vi "Text control 2 v4.5_pump-specific.vi"() -> ()   [LabVIEW 2016]
panel:
  in  "Tab Control":enum32{"Main", "Other parameters"}(tab)
  out "Line running":i32
  out "Total lines":i32
  out "Path":path=path "C:/users/rlp38/09Apr2009LTtesting/test2.txt"
  out "I vs Vg":cluster{"Y data in":dbl[], "X data in":dbl[]}[](graph)
  out "Is":dbl format="%.2e"
  out "Id":dbl format="%.2e"
  out "Ig":dbl format="%.2e"
  out "Id max vs time":cluster{"Y data in":dbl[], "X data in":dbl[]}[](graph)
  out "Id min vs time":cluster{"Y data in":dbl[], "X data in":dbl[]}[](graph)
  out "I vs Vd":cluster{"Y data in":dbl[], "X data in":dbl[]}[](graph)
  in  "Program":string="#pulsedstressV d 0.03 20 0 0.5 0.0827 5\n#\n#itime s\n#gaterangemode l\n#drainrangemode l\n#pump /1Q #query pump\n#wait 1000 #wait 1 second\n#pump /1ZR #initialize pump\n#pump /1Q #query pump\n#wait 20000 #wait 20 seconds\n#pump /1N0R #set step resolution: 0.01 mm\n#pump /1Q #query pump\n#wait 1000 #wait 1 second\n#pump /1V300R #choose speed: 300 steps/s\n#pump /1Q #query pump\n#wait 1000 #wait 1 second\n#pump /1O3R #go to port 3, counterclockwise rotation\n#pump /1Q #query pump\n#wait 1000 #wait 1 second\n#pump /1A2400R #go to absolute position 2400\n#pump /1Q #query pump\n#wait 1000 #wait 1 second\n#pump /1Q #query pump\n#pump /1? #report absolute plunger position\n#pump /1V80R #set speed to 80 steps/s\n#pump /1Q #query pump\n#pump /1O5 #switch to port 5, counterclockwise rotation\n#pump /1Q #query pump\n#wait 200 #wait 200 milliseconds\n#pump /1A0R #go to absolute position 0 (= empty syringe)\n#pump /1Q #query pump\n#pump /1? #report absolute plunger position\n#pulsed on 0.05 0 0.02\n#transfer d 1 -1 -0.1 -1 -1 0\n#wait-min 1\n#transfer d 1 -1 -0.1 -1 -1 0\n#output d 0 -1 -0.5 0 -1 -0.1\n#transfer d -10 40 1 5 40 35\n#transfer d -10 40 1 5 40 35\n#output d 0 40 20 0 40 1\n#\n#\n#sample 1 0.008 221 6 0.003\n#samplei 400e-6 200 6 0.002 0.1\n#vsu2pulse -10 4\n#\n#stressV 0.016 0.03 2e-4 0.1e-3 11\n#stressI 220e-7 0.08 15\n#transfer s -1 1 0.5 -0.005 0.005 0.005\n#output s 0 0 0 -0.008 0.008 0.002"
  out "Command running:":string="#output s 0 0 0 -0.008 0.008 0.002"
  out "Serial port data":string
  out "Elapsed Time":dbl caption="Elapsed Time (s)"
  in  "Units":u16(ring) items=["Seconds", "Minutes", "Hours"]
  in  "Time Offset":dbl caption="Set Start Time (s)"
  in  "Reset":bool
  in  "Auto Reset":bool
  in  "integration time":u32(slide) max=2 step=1 scale=0.0..2.0
  in  "Interrupt run":bool
  out "Absolute plunger position vs time":cluster{"Y data in":dbl[], "X data in":dbl[]}[](graph)
  out "Valve position vs time":cluster{"Y data in":dbl[], "X data in":dbl[]}[](graph)
  in  "Halt pump":bool
  in  "Hard stop pump":bool
  in  "Gate Range\nmode":u16(ring) items=["Auto", "Limited", "Fixed"]
  in  "Gate Range":u8(slide)=6 max=11 scale=0.0..11.0
  in  "Source/Drain\nRange mode":u16(ring) items=["Auto", "Limited", "Fixed"]
  in  "Source/Drain Range":u8(slide)=6 max=11 scale=0.0..11.0
  in  "Panel Controls":T1={"Emergency Stop"=refnum, "TransGraph Max"=1e-05, "Text/Graph (text=false)"=TRUE} {"TransGraph Max" format="%.2e"}
  in  "Panel Controls 2":T2={"Emergency Stop"=refnum, "TransGraph Max"=1e-05, "Text/Graph (text=false)"=TRUE, "TransGraph Min"=1e-11} {"TransGraph Min" format="%.2e"; "TransGraph Max" format="%.2e"}
  in  "SMU4":cluster{"on/off":bool, "Voltage":dbl} {"Voltage" min=-100.0 max=100.0 format="%.2f"}
  in  "Full Reset":bool
  in  "Standby":T3
  out "error out":errorcluster
  in  "Delay before read (ms)":u32=1000
  in  "byte count":u32=64
  in  "Serial End Mode for Reads":u16(ring)=2 items=["None", "LastBit", "TermChar"]
  in  "Timeout (ms)":u32=10000
  in  "Enable Termination\nChar (T)":bool=TRUE
  in  "Termination char\n(0xA = '\\n' = LF)\n(0xD = '\\r' = CR)":u8=13 format="%.0x"
  in  "flow control":u16(ring) items=["None"=0, "XON/XOFF"=1, "RTS/CTS"=2, "DTR/DSR"=4]
  in  "stop bits":u16(ring)=10 items=["1.0"=10, "1.5"=15, "2.0"=20]
  in  "parity":u16(ring) items=["None", "Odd", "Even", "Mark", "Space"]
  in  "data bits":u16=8 min=5 max=8 step=1
  in  "VISA resource name":refnum<visa-resource-name>="COM6"
  in  "baud rate":u32=9600
  in  "Drain: Compliance":dbl=0.001 format="%.8f"
  in  "Gate: Compliance":dbl=0.001 format="%.8f"
  in  "hold time /s":dbl format="%.2f"
  in  "delay time /s":dbl format="%.2f"
  in  "Integration time (short)":dbl=0.0019 min=8e-05 max=0.0019 step=8e-05 format="%^.0e"
  in  "Integration time (long)":dbl=0.32 min=0.04 max=2.0 step=0.02 format="%.2f"
  in  "Step delay /s":dbl format="%.2f"
  in  "Prefix (transfer)":string="_step_1_air_"
  in  "Suffix (transfer)":string="_Vg=0_T_1.txt"
  in  "Prefix (time data)":string="_buffer_Idmax_Idmin_vs_time_Vg=-1.0V_Vd=-1.0V"
  in  "Suffix (time data)":string=".txt"
  in  "Prefix (output)":string="_step_1_air_"
  in  "Suffix (output)":string="_Vg=0_O_1.txt"
  in  "Gate":T4={"Gate Start"=0.0, "Gate Stop"=2.0, "Gate Step (linear only)"=1.0, "Gate Compliance"=0.0001, "Gate PComp"=0.0, "Range mode"=0, "Range"=6} {"Range" max=11 scale=0.0..11.0; "Range mode" items=["Auto", "Limited", "Fixed"]; "Gate PComp" format="%^.2e"; "Gate Compliance" format="%^.2e"; "Gate Step (linear only)" format="%^.4e"; "Gate Stop" format="%^.4e"; "Gate Start" format="%^.4e"}
  in  "Drain 2":T5={"Drain Start"=0.0, "Drain Stop"=2.0, "Drain Compliance"=0.0001, "Drain Step"=1.0, "Drain PComp"=0.0, "Range mode"=0, "Range"=6} {"Range" max=11 scale=0.0..11.0; "Range mode" items=["Auto", "Limited", "Fixed"]; "Drain PComp" format="%^.2e"; "Drain Step" format="%^.4e"; "Drain Compliance" format="%^.2e"; "Drain Stop" format="%^.4e"; "Drain Start" format="%^.4e"}
  in  "Timings 2":T6={"integration time"=0, "Short/Long integration time"=0.00064, "hold time (sec)"=0.0, "delay time (sec)"=0.0, "Step Time (0 disables)"=0.0, "sweep method"=0, "Pulse period"=0.005, "Base voltage"=0.0, "Pulse width"=0.0005} {"Pulse width" min=0.0005 max=0.1 step=0.0001 format="%.4f"; "Base voltage" format="%^.4e"; "Pulse period" min=0.005 max=1.0 step=0.0001 format="%.4f"; "sweep method" items=["Continuous", "Pulsed"]; "Step Time (0 disables)" format="%.2f"; "delay time (sec)" format="%.4f"; "hold time (sec)" format="%.4f"; "Short/Long integration time" format="%^.0e"; "integration time" scale=0.0..2.0}
  # "Syntax:\nitime [s|m|l]\ngaterangemode [a|l|f]\ndrainrangemode [a|l|f]\npulsed [on|off] PulsePeriod(sec) PulseBaseVoltage PulseONWidth(sec)\nstandby [on l off]\nwait NumMilliseconds\nwait-min NumMinutes\n# texthere = comment\ntransfer [s|d] VgStart VgStop VgStep VdStart VdStop VdStep\noutput [s|d] VgStart VgStop VgStep VdStart VdStop VdStep\nsample Vg Vd NumSamples Time(s) SampleInterval(s)\nsamplei Idg NumSamples Time(s) SampleInterval(s) VDGcompliance\n100 samples is approximately 13 seconds with medium integration\n# if in doubt use SampleInterval(s) = 0.004\nstressV VG VD IGcompliance IDcompliance Duration(sec)\nstressI IDG VDGcompliance Duration(sec)\nvsu2pulse Bias Duration(s)\npulsedstressV [s|d] VEstop VgON VgOFF Period(s) PulseONwidth(s) Vd\nsample-fpp Vg Vd NumSamples Time\nresample-fpp Vg Vd\ntransfer-fpp [s|d] VgStart VgStop VgStep VdStart VdStop VdStep\noutput-fpp [s|d] VgStart VgStop VgStep VdStart VdStop VdStep\nserial SerialPortCommand\npump SerialPortCommand for the OEM pump\n\nSPM OEM Pump Syntax (<x>: pump number, use 1 if only one pump):\nif the command syntax contains [R], then append the letter R to the command\n/<x>Q: query (a query command should follow each command)\n/<x>Z[R] or /<x>Y[R]: initialize pump\n/<x>N<n>[R] (<n>=0,1): <0> (<1>) microstep 0.01 mm (0.00125 mm) resolution\n/<x>I<n> (<n>=0-6): turn to port number n (clockwise)\n/<x>O<n> (<n>=0-6): turn to port number n (counterclockwise)\n/<x>X: Re-execute last command string\n/<x>G<n>[R] (<n>=0-60000): repeat command sequence (default: 0, 0=loop forever)\n/<x>g: Mark the start of a repeat sequence (max = 10)\n/<x>M<n>[R] (<n>=0-86400000): delay command execution by n milliseconds\n/<x>H: Halt; Pause the sequence after finishing the current move\n/<x>T: Hardstop; Interrupt the current move and suppress it from the sequence\n/<x>A<n>[R] (<n>=0-3000 with N=0, 0-24000 with N=1): absolute position\n/<x>P<n>[R] (<n>=0-3000 with N=0, 0-24000 with N=1): relative pickup\n/<x>D<n>[R] (<n>=0-3000 with N=0, 0-24000 with N=1): relative dispense\n/<x>V<n>[R] (<n>=5-1600 default: 150): set peak speed (pulses/sec)\n/<x>S<n>[R] (<n>=10-40 default: 22): set speed (NOT in pulses/sec, look in manual)\nNOTE: When controlled with absolute position, one does not need to pay special attention to the syringe that is mounted on the pump.\nWithdraw from lower stage (ports 1, 3, 5), dispense from higher stage (ports 2, 4, 6)."
  # "Time"
  # "1\n2\n3\n4\n5\n6\n7\n8\n9\n10\n11\n12\n13\n14\n15\n16\n17\n18\n19\n20"
  # "Serial port settings"
  # "Filename settings"
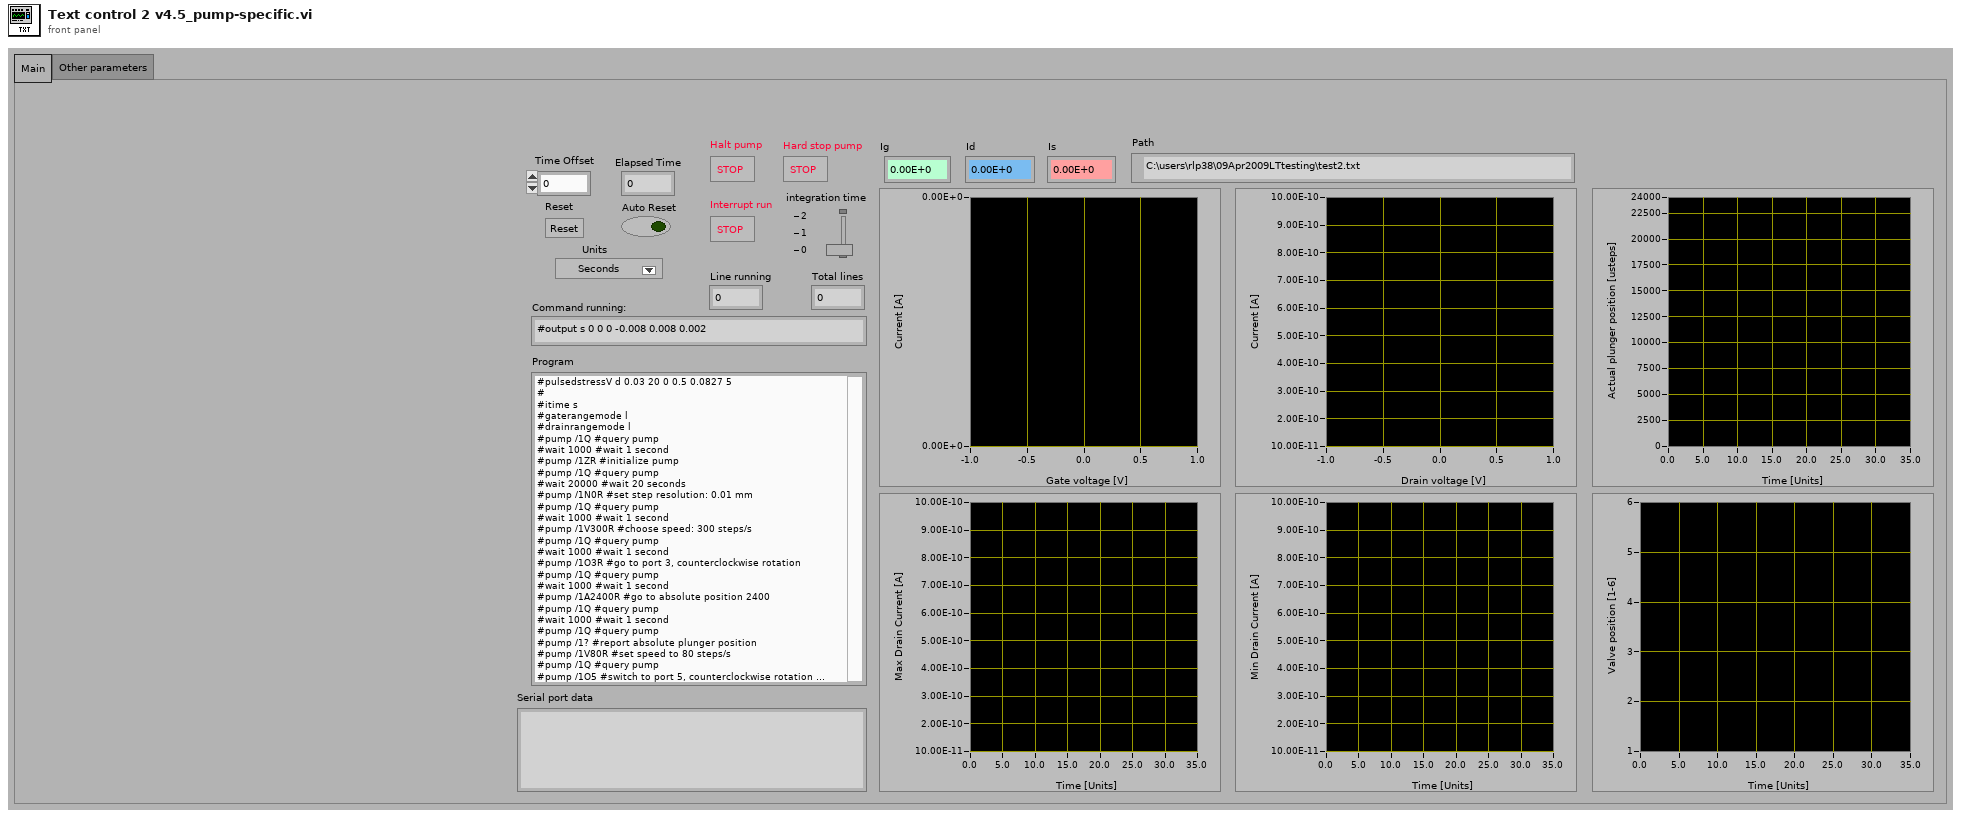
[diagram p1: front panel]
types:
  T1 = cluster{"Emergency Stop":refnum<vi>, "TransGraph Max":dbl, "Text/Graph (text=false)":bool}
  T2 = cluster{"Emergency Stop":refnum<vi>, "TransGraph Max":dbl, "Text/Graph (text=false)":bool, "TransGraph Min":dbl}
  T3 = cluster{"Gate Standby":bool, "Drain Standby":bool}
  T4 = cluster{"Gate Start":dbl, "Gate Stop":dbl, "Gate Step (linear only)":dbl, "Gate Compliance":dbl, "Gate PComp":dbl, "Range mode":u16, "Range":u8}
  T5 = cluster{"Drain Start":dbl, "Drain Stop":dbl, "Drain Compliance":dbl, "Drain Step":dbl, "Drain PComp":dbl, "Range mode":u16, "Range":u8}
  T6 = cluster{"integration time":u32, "Short/Long integration time":dbl, "hold time (sec)":dbl, "delay time (sec)":dbl, "Step Time (0 disables)":dbl, "sweep method":u16, "Pulse period":dbl, "Base voltage":dbl, "Pulse width":dbl}
  T7 = enum16{"open", "replace", "create", "open or create", "replace or create", "replace or create with confirmation"}
  T8 = cluster{"V2 Start":dbl, "V2 Step":dbl, "Number of points":i32}
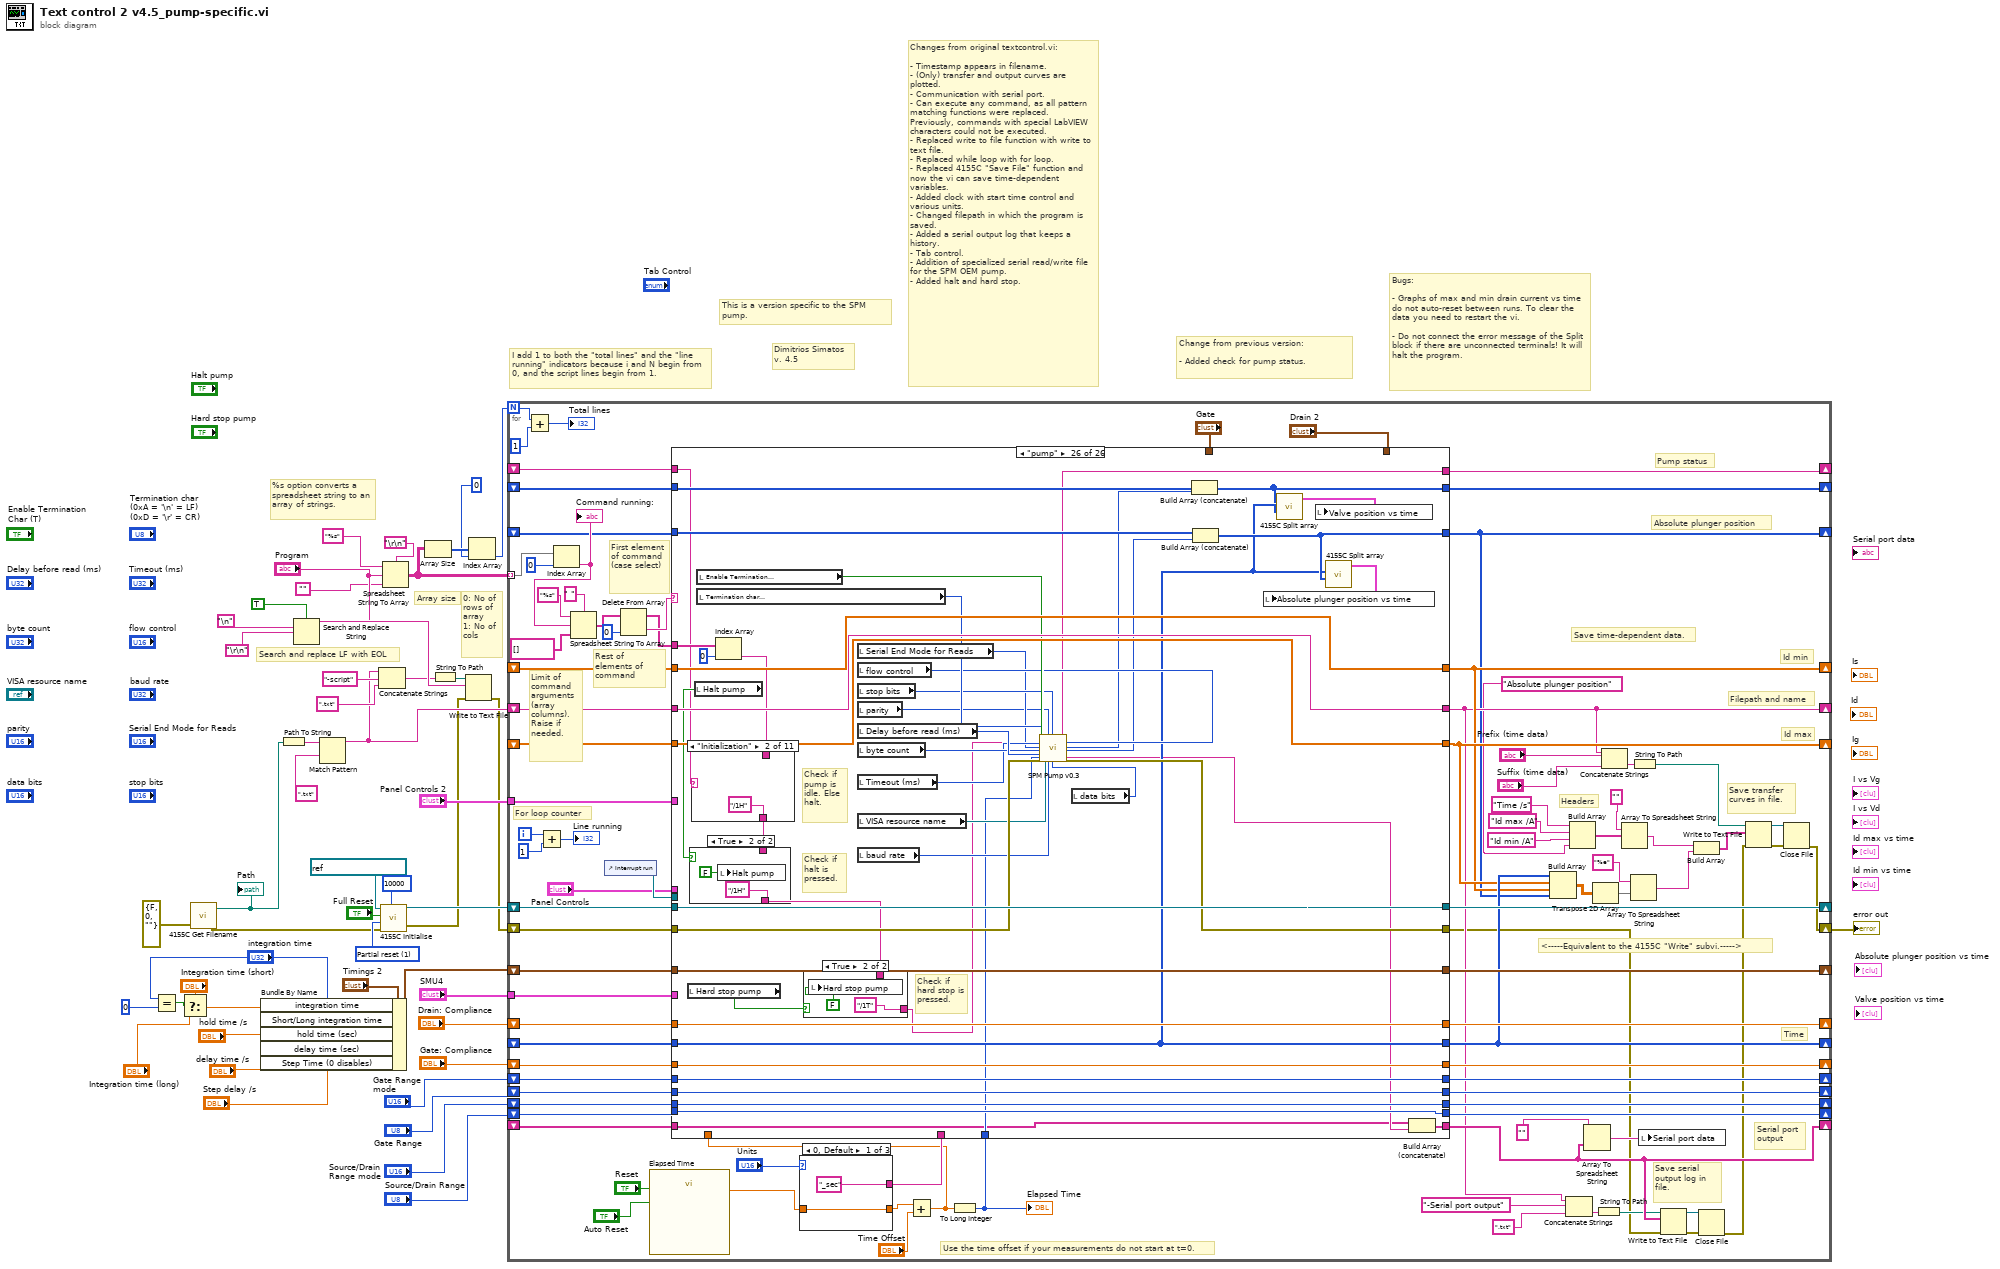
[diagram p0: block diagram]
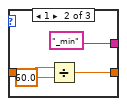
[diagram p2: hidden frame]
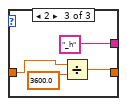
[diagram p3: hidden frame]
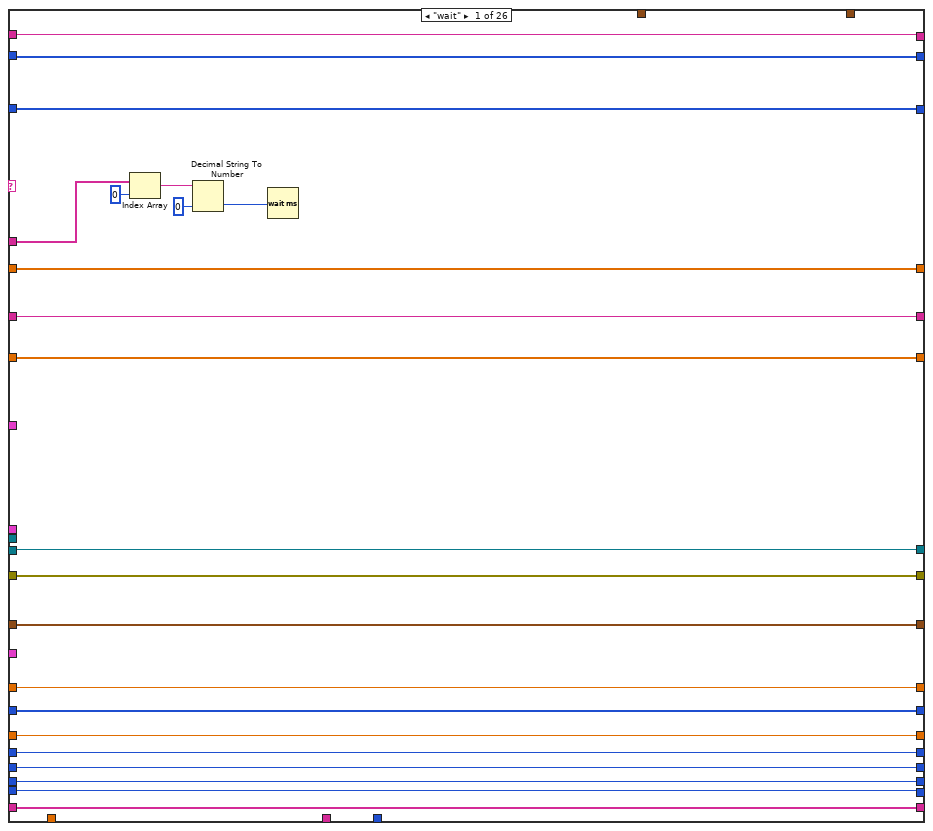
[diagram p4: hidden frame]
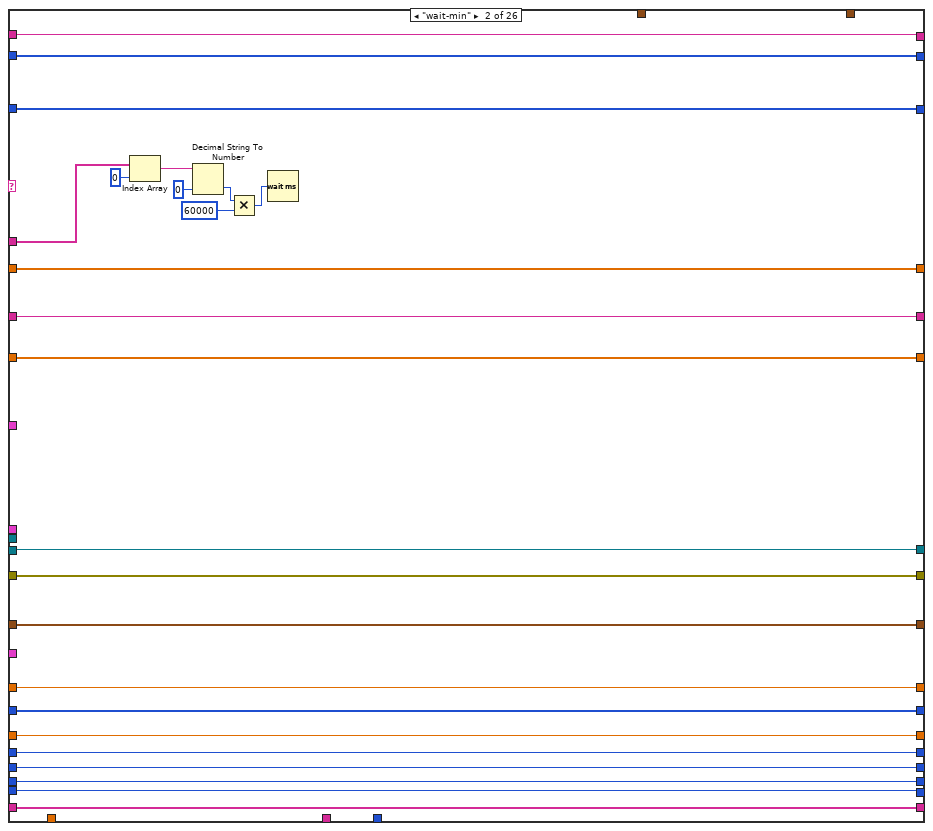
[diagram p5: hidden frame]
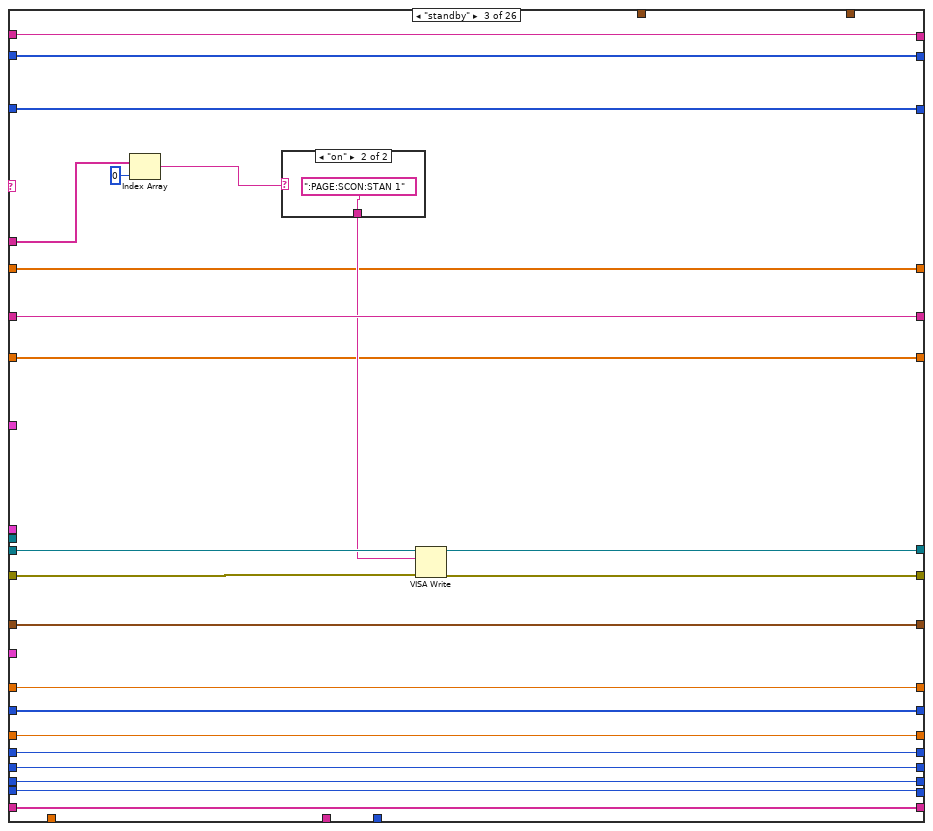
[diagram p6: hidden frame]
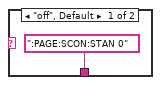
[diagram p7: hidden frame]
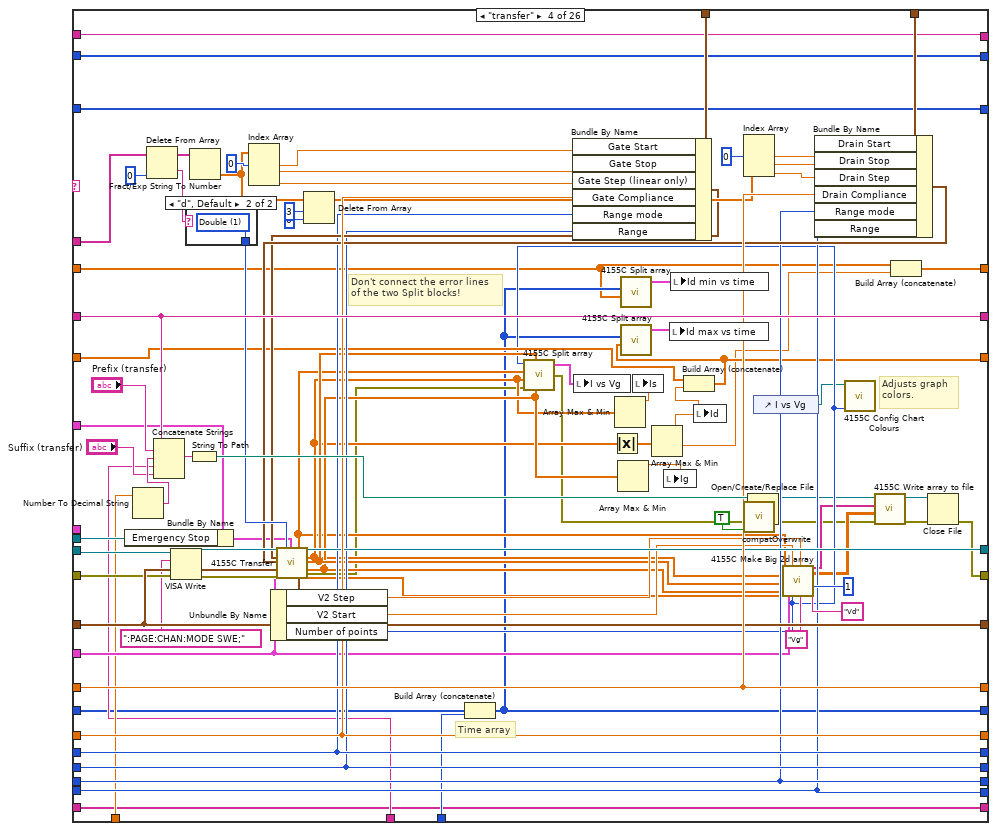
[diagram p8: hidden frame]
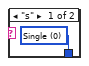
[diagram p9: hidden frame]
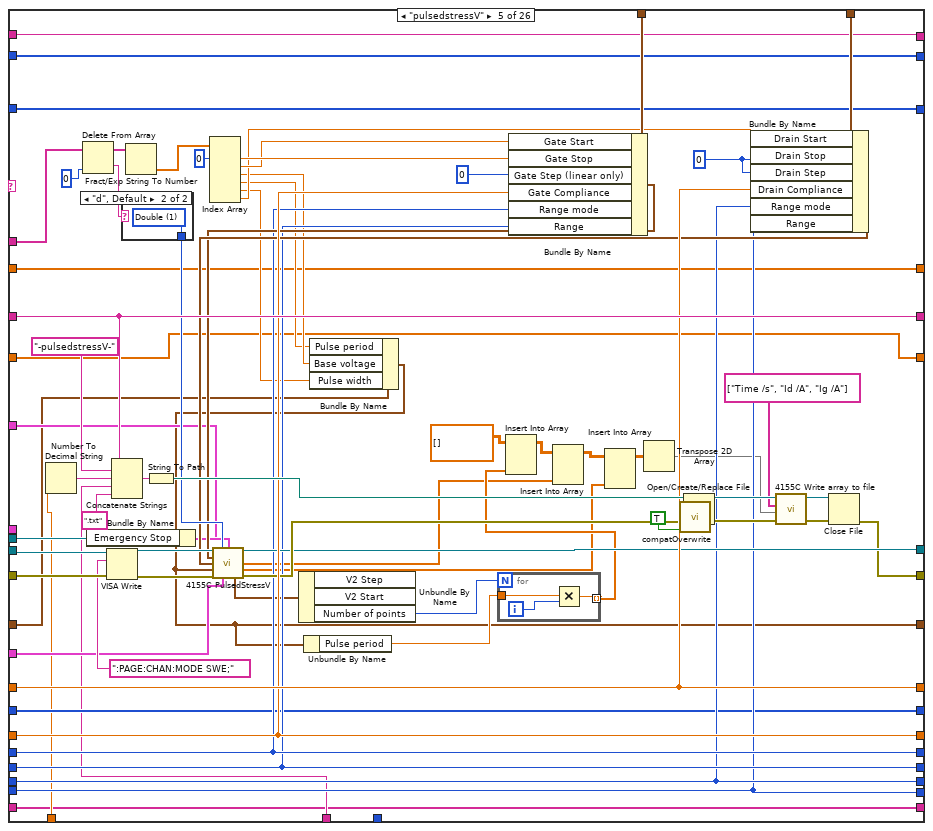
[diagram p10: hidden frame]
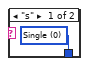
[diagram p11: hidden frame]
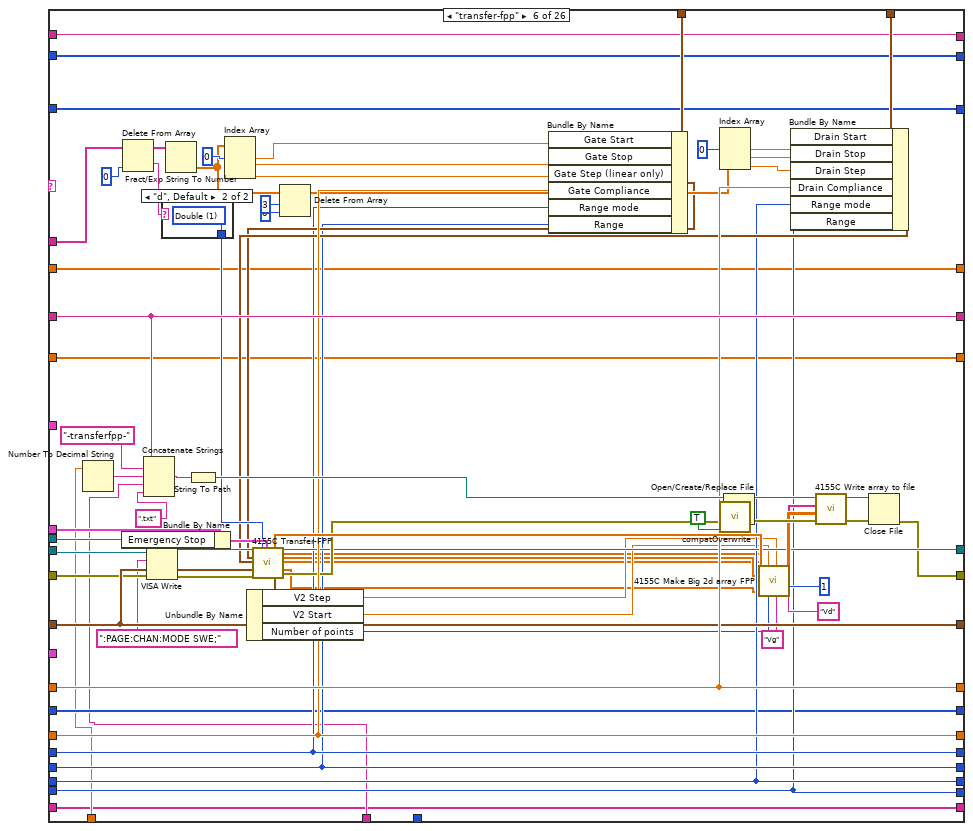
[diagram p12: hidden frame]
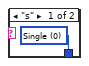
[diagram p13: hidden frame]
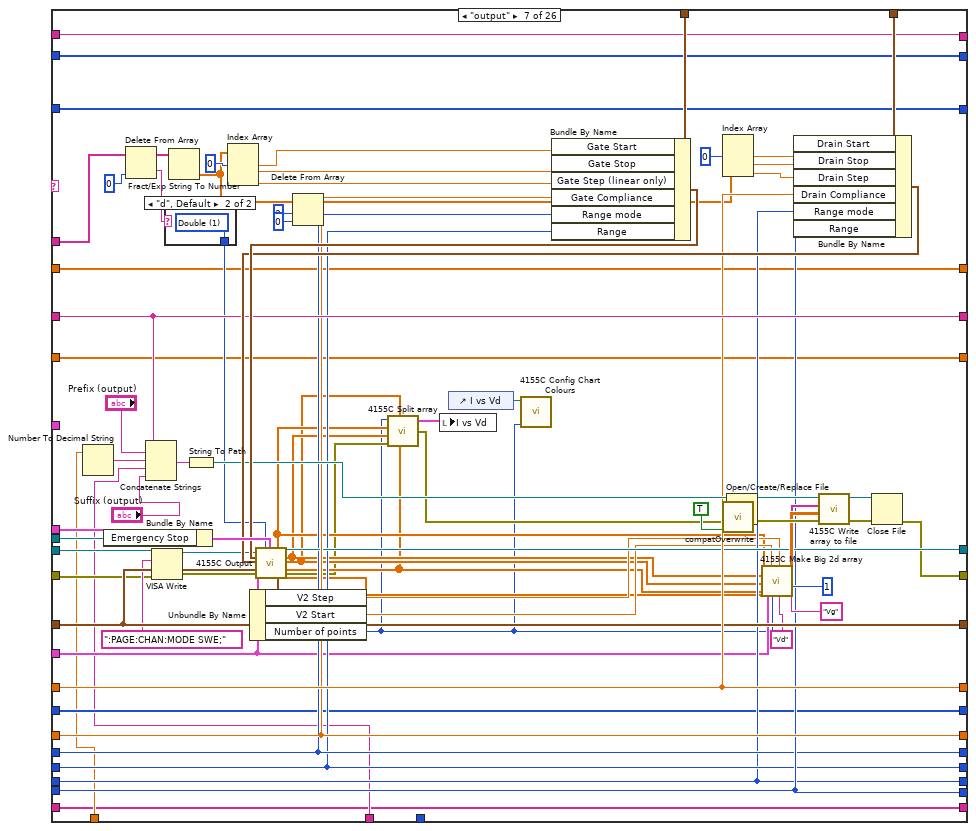
[diagram p14: hidden frame]
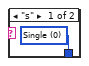
[diagram p15: hidden frame]
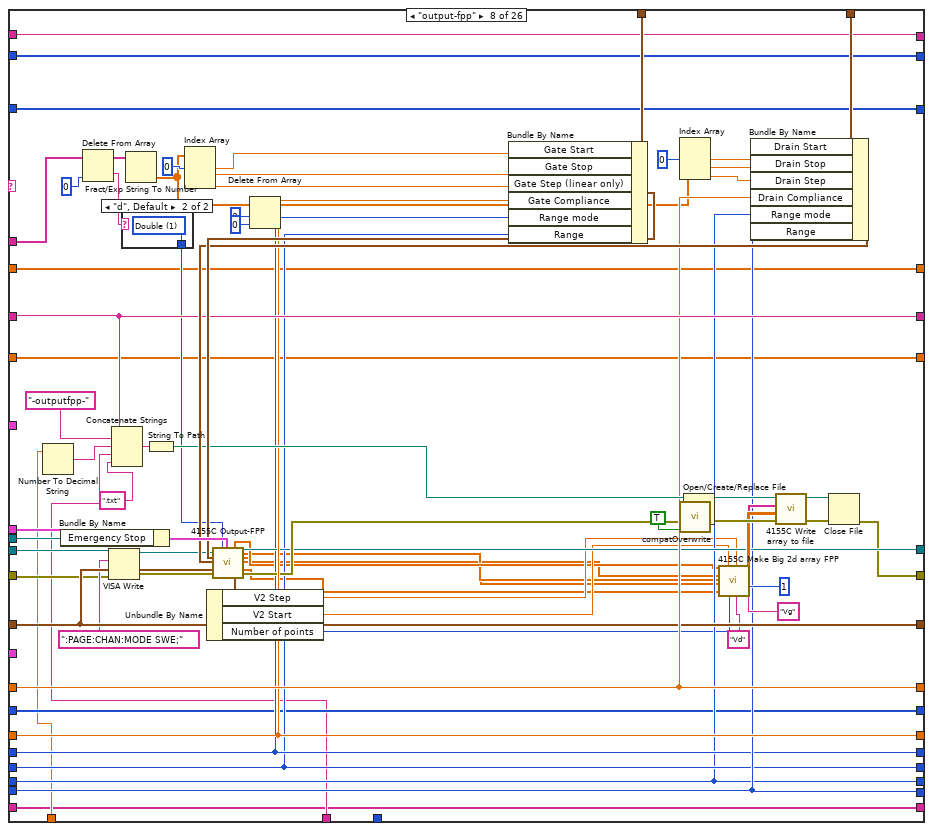
[diagram p16: hidden frame]
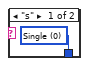
[diagram p17: hidden frame]
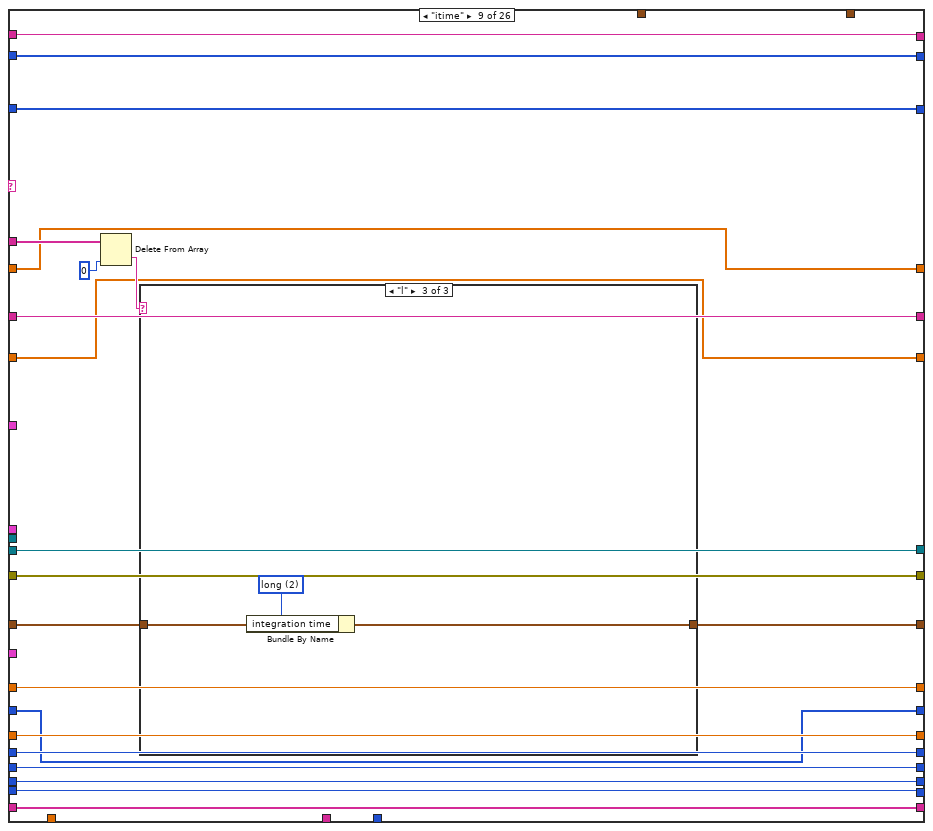
[diagram p18: hidden frame]
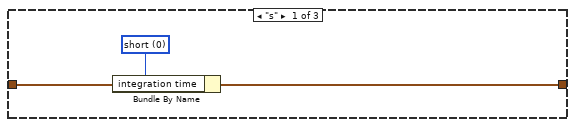
[diagram p19: hidden frame]
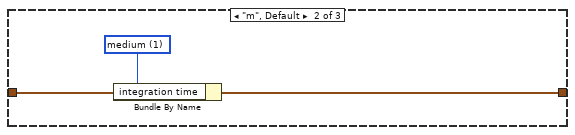
[diagram p20: hidden frame]
diagram:
  w40 = u16 1 items=["Reset All", "Partial reset"] ("Type of reset")
  # "This is a version specific to the SPM pump."
  # "I add 1 to both the \"total lines\" and the \"line running\" indicators because i and N begin from 0, and the script lines begin from 1."
  # "Bugs:\n\n- Graphs of max and min drain current vs time do not auto-reset between runs. To clear the data you need to restart the vi.\n\n- Do not connect the error message of the Split block if there are unconnected terminals! It will halt the program."
  # "Array size"
  # "%s option converts a spreadsheet string to an array of strings."
  # "0: No of rows of array\n1: No of cols"
  # "Change from previous version:\n\n- Added check for pump status."
  # "Dimitrios Simatos\nv. 4.5"
  # "Changes from original textcontrol.vi:\n\n- Timestamp appears in filename.\n- (Only) transfer and output curves are plotted.\n- Communication with serial port.\n- Can execute any command, as all pattern matching functions were replaced. Previously, commands with special LabVIEW characters could not be executed.\n- Replaced write to file function with write to text file.\n- Replaced while loop with for loop.\n- Replaced 4155C \"Save File\" function and now the vi can save time-dependent variables.\n- Added clock with start time control and various units.\n- Changed filepath in which the program is saved.\n- Added a serial output log that keeps a history.\n- Tab control.\n- Addition of specialized serial read/write file for the SPM OEM pump.\n- Added halt and hard stop."
  # "Search and replace LF with EOL"
  n1 = Equal?(x="integration time", y=u32 0) -> (x = y?=w44:bool)
  n2 = Select(t="Integration time (short)", s=w44, f="Integration time (long)") -> (s? t:f=w48:dbl)
  n3 = call "4155C Get Filename.vi"("error in (no error)"=errorcluster {"status"=FALSE, "code"=0, "source"=""}) -> ("error out"=w35:errorcluster, "path"=w10:path)  [unwired: 2 in, 1 out]
  "Path" <- w10
  n4 = Bundle By Name(cluster="Timings 2", "integration time"="integration time", "Short/Long integration time"=w48, "hold time (sec)"="hold time /s", "delay time (sec)"="delay time /s", "Step Time (0 disables)"="Step delay /s") -> (w33:T6)
  n5 = Path To String(path=w10) -> (string=w11:string)
  n6 = Search and Replace String(replace all?=TRUE ("replace all? (F)"), input string="Program", search string="\n", replace string="\r\n") -> (result string=w23:string)  [unwired: 4 in, 3 out]
  n7 = Match Pattern(string=w11, regular expression=".txt") -> (before substring=w5:string)  [unwired: 1 in, 3 out]
  n8 = Concatenate Strings(w5, "-script" ("Prefix"), ".txt" ("regular expression")) -> (w4:string)
  n9 = call "4155C Initialise.vi"("VISA resource name in"=refnum<visa-resource-name> "GPIB0::14::INSTR", "Reset"="Full Reset", "Type of reset"=w40, "error in (no error)"=w35, "VISA Timeout Value"=u32 10000) -> ("VISA Resource Name out"=w34:refnum<visa-resource-name>, "error out"=w2:errorcluster)
  n10 = Spreadsheet String To Array(delimiter (Tab)="\r\n", format string="%s", spreadsheet string="Program", array type (2D Dbl)="") -> (array=w14:string[][])
  n11 = Array Size(array=w14) -> (size(s)=w18:i32[])
  n12 = String To Path(string=w4) -> (path=w3:path)
  n13 = Write to Text File(file (use dialog)=w3, text=w23, error in=w2) -> (error out=w1:errorcluster)  [unwired: 1 in, 2 out]
  n14 = Index Array(array=w18, index=0) -> (element=w16:i32)
  n15 = for {
    N: w16 -> [w75]
    tunnel: "SMU4" -> [w120]
    shift-left: "Source/Drain Range" -> [w125]
    shift-right: [w121] -> _
    shift-left: "Source/Drain\nRange mode" -> [w126]
    shift-right: [w122] -> _
    shift-left: "Gate Range" -> [w127]
    shift-right: [w123] -> _
    shift-left: "Gate Range\nmode" -> [w128]
    shift-right: [w124] -> _
    shift-left: "Gate: Compliance" -> [w137]
    shift-right: [w133] -> _
    shift-left: "Drain: Compliance" -> [w138]
    shift-right: [w134] -> _
    shift-left: w33 -> [w139]
    shift-right: [w135] -> _
    shift-left: w1 -> [w140]
    shift-right: [w83] -> w9
    shift-left: w34 -> [w141]
    shift-right: [w136] -> _
    shift-left: w5 -> [w142]
    shift-right: [w59] -> _
    tunnel: "Panel Controls 2" -> [w119]
    shift-right: [w87] -> _
    shift-left: _ -> [w118]
    shift-right: [w88] -> _
    shift-left: _ -> [w114]
    tunnel: w14 -> [w112] mode=indexing
    shift-right: [w81] -> _
    shift-left: _ -> [w82]
    shift-right: [w64] -> _
    shift-left: _ -> [w67]
    shift-right: [w55] -> _
    shift-left: _ -> [w56]
    shift-right: [w53] -> _
    shift-left: _ -> [w52]
    shift-right: [w51] -> _
    shift-left: _ -> [w50]
    i -> [w70]
    # "Pump status"
    # "Absolute plunger position"
    # "Serial port output"
    # "Save serial output log in file."
    # "For loop counter"
    # "<-----Equivalent to the 4155C \"Write\" subvi.----->"
    # "Headers"
    # "Save transfer curves in file."
    # "Filepath and name"
    # "Save time-dependent data."
    # "Use the time offset if your measurements do not start at t=0."
    # "Time"
    # "Rest of elements of command"
    # "Id min"
    # "Id max"
    # "Limit of command arguments (array columns). Raise if needed."
    # "First element of command\n(case select)"
    n16 = Add(x=w75, y=1) -> (x+y=→"Total lines":i32)
    n17 = Add(x=w70, y=1) -> (x+y=→"Line running":i32)
    n18 = Index Array(array=w112, index=0 ("line index")) -> (element=w107:string)
    "Command running:" <- w107
    n19 = Spreadsheet String To Array(delimiter (Tab)=" ", format string="%s", spreadsheet string=w107, array type (2D Dbl)=string[] []) -> (array=w104:string[])
    n20 = control-ref of="Interrupt run"() -> (w132:refnum<vi>)
    n21 = Delete From Array(array=w104, index=0) -> (deleted portion=w105:string, array with subset deleted=w103:string[])  [unwired: 1 in]
    n22 = call "Elapsed Time"("Reset"="Reset", "Auto Reset"="Auto Reset") -> ("Elapsed Time (s)"=w115:dbl)  [unwired: 10 in, 7 out]
    n23 = case shown="0, Default" "Units" {
      tunnel: ["_sec" "_min" "_h"] -> w116
      tunnel: [w143 w147 w150] -> w77
      tunnel: w115 -> [w143 w146 w151]
      frame 0, Default {
      }
      frame 1 {
        n24 = Divide(x=w146, y=60.0) -> (x/y=w147:dbl)
      }
      frame 2 {
        n25 = Divide(x=w151, y=3600.0) -> (x/y=w150:dbl)
      }
    }
    n26 = Add(x=w77, y="Time Offset") -> (x+y=w76:dbl)
    n27 = To Long Integer(number=w76) -> (32bit integer=w113:i32)
    "Elapsed Time" <- w113
    n28 = case shown="\"pump\"" w105 {
      tunnel: w103 -> [w174 w198 w221 w301 w370 w444 w524 w599 w642 w673 w705 w735 w761 w780 _ _ w899 w965 _ w1040 w1089 w1136 w1211 w1278 w1303 w1352]
      tunnel: w142 -> [w169 w194 w219 w308 w377 w452 w531 w607 w631 w662 w697 w728 w755 w773 w797 w844 w877 w947 w983 w1027 w1076 w1124 w1205 w1274 w1305 w1354]
      tunnel: w141 -> [w168 w193 w210 w279 w361 w421 w500 w575 w632 w663 w698 w729 w756 w774 w802 w846 w905 w971 w987 w1046 w1095 w1142 w1217 w1232 w1309 w1358]
      tunnel: w140 -> [w167 w192 w209 w278 w360 w420 w497 w572 w633 w664 w699 w730 w757 w775 w801 w817 w904 w970 w986 w1045 w1094 w1141 w1216 w1231 w1308 w1357]
      tunnel: w139 -> [w166 w191 w218 w304 w336 w448 w527 w603 w641 w672 w696 w727 w754 w772 w800 w841 w868 w939 w992 w1020 w1069 w1117 w1204 w1273 w1310 w1359]
      tunnel: w138 -> [w165 w190 w217 w306 w375 w450 w529 w605 w640 w671 w704 w734 w760 w779 w799 w826 w903 w969 w995 w1044 w1093 w1140 w1215 w1282 w1311 w1360]
      tunnel: w137 -> [w164 w189 w216 w305 w374 w449 w528 w604 w639 w670 w703 w733 w759 w778 w798 w827 w878 w948 w994 w1028 w1077 w1125 w1206 w1275 w1313 w1361]
      tunnel: [w168 w193 w208 w303 w372 w446 w526 w601 w632 w663 w698 w729 w756 w774 w802 w846 w869 w921 w985 w1021 w1070 w1118 w1157 w1234 w1309 w1358] -> w136
      tunnel: [w167 w192 w207 w302 w371 w445 w525 w600 w633 w664 w699 w730 w757 w775 w801 w816 w879 w922 w984 w1029 w1078 w1126 w1156 w1233 w1307 w1356] -> w58
      tunnel: [w166 w191 w218 w304 w332 w448 w527 w603 w634 w665 w696 w727 w754 w772 w800 w841 w868 w939 w992 w1020 w1069 w1117 w1204 w1273 w1310 w1359] -> w135
      tunnel: [w165 w190 w217 w306 w375 w450 w529 w605 w640 w671 w704 w734 w760 w779 w799 w826 w903 w969 w995 w1044 w1093 w1140 w1215 w1282 w1311 w1360] -> w134
      tunnel: [w164 w189 w216 w305 w374 w449 w528 w604 w639 w670 w703 w733 w759 w778 w798 w827 w878 w948 w994 w1028 w1077 w1125 w1206 w1275 w1313 w1361] -> w133
      tunnel: [w169 w194 w219 w308 w377 w452 w531 w607 w631 w662 w697 w728 w755 w773 w797 w844 w877 w947 w983 w1027 w1076 w1124 w1205 w1274 w1305 w1354] -> w59
      tunnel: w132 -> [_ _ _ w311 w381 w457 w535 w611 _ _ _ _ _ _ _ _ w874 w944 _ w1026 w1075 w1123 w1177 w1250 _ _]
      tunnel: "Gate" -> [_ _ _ w288 w364 w431 w511 w586 _ _ _ _ _ _ _ _ _ _ _ _ _ _ _ _ _ _]
      tunnel: "Drain 2" -> [_ _ _ w287 w363 w430 w510 w585 _ _ _ _ _ _ _ _ _ _ _ _ _ _ _ _ _ _]
      tunnel: "Panel Controls" -> [_ _ _ _ _ w429 w509 w584 _ _ _ _ _ _ _ _ _ _ _ _ _ _ _ _ _ _]
      tunnel: w128 -> [w163 w188 w215 w272 w354 w414 w495 w570 w638 w669 _ w726 w753 w771 w796 w828 w864 w935 w988 w1016 w1065 w1113 w1200 w1269 w1314 w1362]
      tunnel: w127 -> [w162 w187 w214 w271 w353 w413 w494 w569 w637 w668 w702 _ w744 w777 w795 w829 w865 w936 w989 w1017 w1066 w1114 w1201 w1270 w1315 w1363]
      tunnel: w126 -> [w161 w186 w213 w270 w352 w412 w493 w568 w636 w667 w701 w732 w758 _ w794 w830 w866 w937 w990 w1018 w1067 w1115 w1202 w1271 w1316 w1364]
      tunnel: w125 -> [w160 w185 w212 w269 w351 w411 w496 w571 w635 w666 w700 w731 _ w776 w793 w831 w867 w938 w991 w1019 w1068 w1116 w1203 w1272 w1317 w1365]
      tunnel: [w163 w188 w215 w272 w354 w414 w495 w570 w638 w669 w695 w726 w753 w771 w796 w828 w864 w935 w988 w1016 w1065 w1113 w1200 w1269 w1314 w1362] -> w124
      tunnel: [w162 w187 w214 w271 w353 w413 w494 w569 w637 w668 w702 w718 w744 w777 w795 w829 w865 w936 w989 w1017 w1066 w1114 w1201 w1270 w1315 w1363] -> w123
      tunnel: [w161 w186 w213 w270 w352 w412 w493 w568 w636 w667 w701 w732 w758 w770 w794 w830 w866 w937 w990 w1018 w1067 w1115 w1202 w1271 w1316 w1364] -> w122
      tunnel: [w160 w185 w212 w269 w351 w411 w496 w571 w635 w666 w700 w731 w745 w776 w793 w831 w867 w938 w991 w1019 w1068 w1116 w1203 w1272 w1317 w1365] -> w121
      tunnel: w120 -> [_ _ _ w264 w348 _ w489 _ _ _ _ _ _ _ _ _ _ _ _ _ _ _ _ _ _ _]
      tunnel: w119 -> [_ _ _ w262 w347 _ _ _ _ _ _ _ _ _ _ _ _ _ _ _ _ _ _ _ _ _]
      tunnel: [w159 w181 w205 w239 w324 w401 w486 w557 w630 w660 w694 w717 w743 w769 w792 w812 w856 w919 w982 w1005 w1058 w1107 w1154 w1227 w1306 w1355] -> w87
      tunnel: w118 -> [w159 w181 w205 w253 w324 w401 w486 w557 w630 w660 w694 w717 w743 w769 w792 w812 w856 w919 w982 w1005 w1058 w1107 w1154 w1227 w1306 w1355]
      tunnel: w76 -> [_ _ _ w249 w321 w399 w483 w554 _ _ _ _ _ _ _ w810 w854 w916 _ w1002 w1055 w1104 w1151 w1223 _ _]
      tunnel: w116 -> [_ _ _ w246 w320 w397 w482 w553 _ _ _ _ _ _ _ w808 w852 w915 _ w1001 w1054 w1103 w1150 w1224 _ _]
      tunnel: w113 -> [_ _ _ w240 _ _ _ _ _ _ _ _ _ _ _ _ _ _ _ _ _ _ _ _ _ w1320]
      tunnel: [w158 w180 w204 w237 w323 w400 w485 w556 w629 w659 w693 w716 w742 w768 w791 w811 w855 w918 w981 w1004 w1057 w1106 w1153 w1226 w1312 w1334] -> w88
      tunnel: w114 -> [w158 w180 w204 w245 w323 w400 w485 w556 w629 w659 w693 w716 w742 w768 w791 w811 w855 w918 w981 w1004 w1057 w1106 w1153 w1226 w1312 w1334]
      tunnel: [w157 w179 w203 w235 w319 w396 w481 w552 w628 w658 w692 w715 w741 w767 w790 w807 w851 w914 w980 w1000 w1053 w1102 w1149 w1222 w1301 w1351] -> w81
      tunnel: w82 -> [w157 w179 w203 w234 w319 w396 w481 w552 w628 w658 w692 w715 w741 w767 w790 w807 w851 w914 w980 w1000 w1053 w1102 w1149 w1222 w1301 w1351]
      tunnel: [w156 w178 w202 w227 w318 w395 w471 w551 w627 w657 w691 w714 w740 w766 w789 w806 w850 w913 w979 w999 w1052 w1101 w1148 w1221 w1300 w1350] -> w64
      tunnel: w67 -> [w156 w178 w202 w227 w318 w395 w471 w551 w627 w657 w691 w714 w740 w766 w789 w806 w850 w913 w979 w999 w1052 w1101 w1148 w1221 w1299 w1318]
      tunnel: [w155 w177 w201 w226 w317 w394 w470 w550 w626 w656 w690 w713 w739 w765 w788 w805 w849 w912 w978 w998 w1051 w1100 w1147 w1220 w1285 w1336] -> w55
      tunnel: w56 -> [w155 w177 w201 w226 w317 w394 w470 w550 w626 w656 w690 w713 w739 w765 w788 w805 w849 w912 w978 w998 w1051 w1100 w1147 w1220 w1285 w1335]
      tunnel: [w154 w176 w200 w225 w316 w393 w469 w549 w625 w655 w689 w712 w738 w764 w787 w804 w848 w911 w977 w997 w1050 w1099 w1146 w1219 w1284 w1332] -> w53
      tunnel: w52 -> [w154 w176 w200 w225 w316 w393 w469 w549 w625 w655 w689 w712 w738 w764 w787 w804 w848 w911 w977 w997 w1050 w1099 w1146 w1219 w1284 w1331]
      tunnel: [w153 w175 w199 w224 w315 w392 w468 w548 w624 w654 w688 w711 w737 w763 w786 w803 w847 w910 w976 w996 w1049 w1098 w1145 w1218 w1283 w1322] -> w51
      tunnel: w50 -> [w153 w175 w199 w224 w315 w392 w468 w548 w624 w654 w688 w711 w737 w763 w786 w803 w847 w910 w976 w996 w1049 w1098 w1145 w1218 w1283 w1321]
      frame "wait" {
        n29 = Index Array(array=w174, index=0 ("Index")) -> (element=w172:string)
        n30 = Decimal String To Number(string=w172, default (0L)=u32 0) -> (number=w171:u32)  [unwired: 1 in, 1 out]
        n31 = Wait (ms)(milliseconds to wait=w171) -> ()  [unwired: 1 out]
      }
      frame "wait-min" {
        n32 = Index Array(array=w198, index=0 ("Index")) -> (element=w196:string)
        n33 = Decimal String To Number(string=w196, default (0L)=u32 0) -> (number=w184:u32)  [unwired: 1 in, 1 out]
        n34 = Multiply(x=w184, y=u32 60000) -> (x*y=w183:u32)
        n35 = Wait (ms)(milliseconds to wait=w183) -> ()  [unwired: 1 out]
      }
      frame "standby" {
        n36 = Index Array(array=w221, index=0 ("Index")) -> (element=w211:string)
        n37 = case shown="\"on\"" w211 {
          tunnel: [":PAGE:SCON:STAN 0" ":PAGE:SCON:STAN 1"] -> w206
          frame "off", Default {
          }
          frame "on" {
          }
        }
        n38 = VISA Write(VISA resource name=w210, write buffer=w206, error in (no error)=w209) -> (VISA resource name out=w208:refnum<visa-resource-name>, error out=w207:errorcluster)  [unwired: 1 out]
      }
      frame "transfer" {
        # "Don't connect the error lines\nof the two Split blocks!"
        # "Adjusts graph colors."
        # "Time array"
        n39 = Bundle By Name(cluster=w262, "Emergency Stop"=w311) -> (w263:T2)
        n40 = Number To Decimal String(number=w249) -> (decimal integer string=w248:string)  [unwired: 1 in]
        n41 = Delete From Array(array=w301, index=0 ("Index")) -> (deleted portion=w299:string, array with subset deleted=w298:string[])  [unwired: 1 in]
        n42 = Concatenate Strings(w308, "Prefix (transfer)", w248, w246, "Suffix (transfer)") -> (w310:string)
        n43 = VISA Write(VISA resource name=w279, write buffer=":PAGE:CHAN:MODE SWE;" ("write buffer (\"\")"), error in (no error)=w278) -> (VISA resource name out=w276:refnum<visa-resource-name>, error out=w277:errorcluster)  [unwired: 1 out]
        n44 = case shown="\"d\", Default" w299 {
          tunnel: [w313 w314] -> w297
          frame "s" {
            w313 = u16 0 items=["Single", "Double"] ("sweep mode")
          }
          frame "d", Default {
            w314 = u16 1 items=["Single", "Double"] ("sweep mode")
          }
        }
        n45 = String To Path(string=w310) -> (path=w307:path)
        n46 = Fract/Exp String To Number(string=w298) -> (number=w283:dbl[])  [unwired: 3 in, 1 out]
        n47 = Index Array(array=w283, index #1=0 ("Index")) -> (element #1=w296:dbl, element #2=w295:dbl, element #3=w294:dbl)  [unwired: 2 in]
        n48 = Delete From Array(array=w283, length=3 ("Length"), index=0 ("Index")) -> (array with subset deleted=w281:dbl[])  [unwired: 1 out]
        n49 = Build Array (concatenate)(w245, w240) -> (w237:i32[])
        n50 = Bundle By Name(cluster=w288, "Gate Start"=w296, "Gate Stop"=w295, "Gate Step (linear only)"=w294, "Gate Compliance"=w305, "Range mode"=w272, "Range"=w271) -> (w273:T4)
        n51 = call "4155C Split array.vi"("X data in"=w237, "Y1 data in"=w234) -> ("Array of clusters"=w238:cluster{"Y data in":dbl[], "X data in":dbl[]}[])  [unwired: 5 in, 1 out]
        n52 = local write "Id min vs time"(w238) -> ()
        n53 = Index Array(array=w281, index #1=0 ("Index")) -> (element #1=w291:dbl, element #2=w290:dbl, element #3=w289:dbl)  [unwired: 2 in]
        n54 = call <vilib>:"compatOverwrite.vi"("overwrite (F)"=TRUE) -> ("overwrite?"=w261:T7)
        n55 = control-ref of="I vs Vg"() -> (w250:refnum<vi>)
        n56 = Bundle By Name(cluster=w287, "Drain Start"=w291, "Drain Stop"=w290, "Drain Step"=w289, "Drain Compliance"=w306, "Range mode"=w270, "Range"=w269) -> (w274:T5)
        n57 = call "4155C Transfer.vi"("VISA resource name in"=w276, "Gate"=w273, "Drain"=w274, "Timings"=w304, "error in (no error)"=w277, "SMU4"=w264, "sweep mode"=w297, "Panel Controls"=w263) -> ("VG"=w254:dbl[], "Outparams"=w268:T8, "VISA Resource Name out"=w303:refnum<visa-resource-name>, "IS"=w255:dbl[], "ID"=w260:dbl[], "IG"=w256:dbl[], "error out"=w241:errorcluster, "SMU4"=w265:dbl[])  [unwired: 12 in]
        n58 = Unbundle By Name(w268) -> ("V2 Step"=w267:dbl, "V2 Start"=w266:dbl, "Number of points"=w251:i32)
        n59 = call "4155C Split array.vi"("Number of VAR2 steps"=w251, "Y2 data in"=w260, "X data in"=w254, "Y1 data in"=w255, "Y3 data in"=w256, "error in (no error)"=w241) -> ("Array of clusters"=w244:cluster{"Y data in":dbl[], "X data in":dbl[]}[], "error out"=w242:errorcluster)  [unwired: 1 in]
        n60 = local write "I vs Vg"(w244) -> ()
        n61 = Absolute Value(x=w255) -> (abs(x)=w259:dbl[])
        n62 = Array Max & Min(array=w255) -> (max value=w257:dbl)  [unwired: 3 out]
        n63 = Array Max & Min(array=w256) -> (max value=w258:dbl)  [unwired: 3 out]
        n64 = local write "Is"(w257) -> ()
        n65 = Array Max & Min(array=w259) -> (max value=w252:dbl, min value=w236:dbl)  [unwired: 2 out]
        n66 = local write "Ig"(w258) -> ()
        n67 = Build Array (concatenate)(w253, w252) -> (w239:dbl[])
        n68 = call "4155C Split array.vi"("X data in"=w237, "Y1 data in"=w239) -> ("Array of clusters"=w243:cluster{"Y data in":dbl[], "X data in":dbl[]}[])  [unwired: 5 in, 1 out]
        n69 = local write "Id max vs time"(w243) -> ()
        n70 = local write "Id"(w252) -> ()
        n71 = Open/Create/Replace File(file path (use dialog)=w307, error in=w242, operation (0:open)=w261) -> (refnum out=w232:refnum<file>, error out=w230:errorcluster)  [unwired: 3 in, 1 out]
        n72 = call "4155C Make Big 2d array.vi"("1D Var1"=w254, "1d IS"=w255, "1d ID"=w260, "1d IG"=w256, "1d SMU4"=w265, "SMU4"=w264, "VAR2 START"=w266, "Number of VAR2 steps"=w251, "VAR2 STEP"=w267, "VAR1 Name"="Vg", "Decimal places in header"=i8 1, "VAR2 Name"="Vd") -> ("Header array"=w233:string[], "Data array"=w231:dbl[][])  [unwired: 14 in]
        n73 = call "4155C Config Chart Colours.vi"("Numeric"=w251, "XY Graph 2"=w250) -> ()  [unwired: 6 in]
        n74 = call "4155C Write array to file.vi"("Byte Stream File Refnum"=w232, "Header"=w233, "Data Array"=w231, "error in (no error)"=w230) -> ("dup refnum"=w229:refnum<file>, "error out"=w228:errorcluster)  [unwired: 1 in]
        n75 = Build Array (concatenate)(w234, w236) -> (w235:dbl[])
        n76 = Close File(refnum=w229, error in=w228) -> (error out=w302:errorcluster)  [unwired: 1 out]
      }
      frame "pulsedstressV" {
        w330 = 0
        n77 = Number To Decimal String(number=w321) -> (decimal integer string=w378:string)  [unwired: 1 in]
        n78 = Delete From Array(array=w370, index=0 ("Index")) -> (deleted portion=w368:string, array with subset deleted=w367:string[])  [unwired: 1 in]
        n79 = Bundle By Name(cluster=w347, "Emergency Stop"=w381) -> (w349:T2)
        n80 = VISA Write(VISA resource name=w361, write buffer=":PAGE:CHAN:MODE SWE;" ("write buffer (\"\")"), error in (no error)=w360) -> (VISA resource name out=w358:refnum<visa-resource-name>, error out=w359:errorcluster)  [unwired: 1 out]
        n81 = Concatenate Strings(w377, "-pulsedstressV-" ("Substring"), w378, w320, ".txt" ("Substring")) -> (w380:string)
        n82 = case shown="\"d\", Default" w368 {
          tunnel: [w390 w391] -> w366
          frame "s" {
            w390 = u16 0 items=["Single", "Double"] ("sweep mode")
          }
          frame "d", Default {
            w391 = u16 1 items=["Single", "Double"] ("sweep mode")
          }
        }
        n83 = Fract/Exp String To Number(string=w367) -> (number=w362:dbl[])  [unwired: 3 in, 1 out]
        n84 = String To Path(string=w380) -> (path=w376:path)
        n85 = Index Array(array=w362, index #1=0 ("Index")) -> (element #1=w339:dbl, element #2=w338:dbl, element #3=w335:dbl, element #4=w334:dbl, element #5=w333:dbl, element #6=w337:dbl)  [unwired: 5 in]
        n86 = Bundle By Name(cluster=w336, "Pulse period"=w334, "Base voltage"=w335, "Pulse width"=w333) -> (w332:T6)
        n87 = Unbundle By Name(w332) -> ("Pulse period"=w340:dbl)
        n88 = Bundle By Name(cluster=w364, "Gate Start"=w338, "Gate Stop"=w339, "Gate Step (linear only)"=0, "Gate Compliance"=w374, "Range mode"=w354, "Range"=w353) -> (w355:T4)
        n89 = call <vilib>:"compatOverwrite.vi"("overwrite (F)"=TRUE) -> ("overwrite?"=w325:T7)
        n90 = Bundle By Name(cluster=w363, "Drain Start"=w337, "Drain Stop"=w330, "Drain Step"=w330, "Drain Compliance"=w375, "Range mode"=w352, "Range"=w351) -> (w356:T5)
        n91 = call "4155C PulsedStressV.vi"("VISA resource name in"=w358, "sweep mode"=w366, "Panel Controls"=w349, "Gate"=w355, "Drain"=w356, "Timings"=w332, "error in (no error)"=w359, "SMU4"=w348) -> ("VISA Resource Name out"=w372:refnum<visa-resource-name>, "ID"=w328:dbl[], "IG"=w326:dbl[], "Outparams"=w350:T8, "error out"=w373:errorcluster)  [unwired: 3 in]
        n92 = Unbundle By Name(w350) -> ("Number of points"=w327:i32)  [unwired: 2 out]
        n93 = for {
          N: w327 -> [_]
          tunnel: [w387] -> w329 mode=indexing
          tunnel: w340 -> [w389]
          i -> [w388]
          n94 = Multiply(x=w389, y=w388) -> (x*y=w387:dbl)
        }
        n95 = Insert Into Array(array=dbl[][] [] ("Input Array"), new element=w329) -> (w341:dbl[][])  [unwired: 2 in]
        n96 = Insert Into Array(array=w341, new element=w328) -> (w346:dbl[][])  [unwired: 2 in]
        n97 = Insert Into Array(array=w346, new element=w326) -> (w345:dbl[][])  [unwired: 2 in]
        n98 = Transpose 2D Array(2D array=w345) -> (transposed array=w344:dbl[][])
        n99 = Open/Create/Replace File(file path (use dialog)=w376, error in=w373, operation (0:open)=w325) -> (refnum out=w384:refnum<file>, error out=w385:errorcluster)  [unwired: 3 in, 1 out]
        n100 = call "4155C Write array to file.vi"("Byte Stream File Refnum"=w384, "Header"=string[] ["Time /s", "Id /A", "Ig /A"], "Data Array"=w344, "error in (no error)"=w385) -> ("dup refnum"=w382:refnum<file>, "error out"=w383:errorcluster)  [unwired: 1 in]
        n101 = Close File(refnum=w382, error in=w383) -> (error out=w371:errorcluster)  [unwired: 1 out]
      }
      frame "transfer-fpp" {
        n102 = Number To Decimal String(number=w399) -> (decimal integer string=w453:string)  [unwired: 1 in]
        n103 = Bundle By Name(cluster=w429, "Emergency Stop"=w457) -> (w465:T1)
        n104 = Delete From Array(array=w444, index=0 ("Index")) -> (deleted portion=w442:string, array with subset deleted=w441:string[])  [unwired: 1 in]
        n105 = Concatenate Strings(w452, "-transferfpp-" ("Substring"), w453, w397, ".txt" ("Substring")) -> (w455:string)
        n106 = VISA Write(VISA resource name=w421, write buffer=":PAGE:CHAN:MODE SWE;" ("write buffer (\"\")"), error in (no error)=w420) -> (VISA resource name out=w418:refnum<visa-resource-name>, error out=w419:errorcluster)  [unwired: 1 out]
        n107 = case shown="\"d\", Default" w442 {
          tunnel: [w466 w467] -> w440
          frame "s" {
            w466 = u16 0 items=["Single", "Double"] ("sweep mode")
          }
          frame "d", Default {
            w467 = u16 1 items=["Single", "Double"] ("sweep mode")
          }
        }
        n108 = Fract/Exp String To Number(string=w441) -> (number=w425:dbl[])  [unwired: 3 in, 1 out]
        n109 = String To Path(string=w455) -> (path=w451:path)
        n110 = Index Array(array=w425, index #1=0 ("Index")) -> (element #1=w439:dbl, element #2=w438:dbl, element #3=w437:dbl)  [unwired: 2 in]
        n111 = Delete From Array(array=w425, length=3 ("Length"), index=0 ("Index")) -> (array with subset deleted=w423:dbl[])  [unwired: 1 out]
        n112 = Bundle By Name(cluster=w431, "Gate Start"=w439, "Gate Stop"=w438, "Gate Step (linear only)"=w437, "Gate Compliance"=w449, "Range mode"=w414, "Range"=w413) -> (w415:T4)
        n113 = Index Array(array=w423, index #1=0 ("Index")) -> (element #1=w434:dbl, element #2=w433:dbl, element #3=w432:dbl)  [unwired: 2 in]
        n114 = call <vilib>:"compatOverwrite.vi"("overwrite (F)"=TRUE) -> ("overwrite?"=w402:T7)
        n115 = Bundle By Name(cluster=w430, "Drain Start"=w434, "Drain Stop"=w433, "Drain Step"=w432, "Drain Compliance"=w450, "Range mode"=w412, "Range"=w411) -> (w416:T5)
        n116 = call "4155C Transfer-FPP.vi"("VISA resource name in"=w418, "Gate"=w415, "Drain"=w416, "Timings"=w448, "error in (no error)"=w419, "sweep mode"=w440, "Panel Controls"=w465) -> ("VG"=w456:dbl[], "Outparams"=w410:T8, "VISA Resource Name out"=w446:refnum<visa-resource-name>, "Vprobe2"=w406:dbl[], "ID"=w405:dbl[], "IG"=w404:dbl[], "Vprobe1"=w403:dbl[], "error out"=w447:errorcluster)  [unwired: 13 in]
        n117 = Unbundle By Name(w410) -> ("V2 Step"=w409:dbl, "V2 Start"=w408:dbl, "Number of points"=w407:i32)
        n118 = Open/Create/Replace File(file path (use dialog)=w451, error in=w447, operation (0:open)=w402) -> (refnum out=w462:refnum<file>, error out=w463:errorcluster)  [unwired: 3 in, 1 out]
        n119 = call "4155C Make Big 2d array FPP.vi"("1D Var1"=w456, "1d ID"=w405, "1d Vp2"=w406, "1d IG"=w404, "1d Vp1"=w403, "VAR2 START"=w408, "Number of VAR2 steps"=w407, "VAR2 STEP"=w409, "VAR1 Name"="Vg", "Decimal places in header"=i8 1, "VAR2 Name"="Vd") -> ("Header array"=w458:string[], "Data array"=w459:dbl[][])  [unwired: 15 in]
        n120 = call "4155C Write array to file.vi"("Byte Stream File Refnum"=w462, "Header"=w458, "Data Array"=w459, "error in (no error)"=w463) -> ("dup refnum"=w460:refnum<file>, "error out"=w461:errorcluster)  [unwired: 1 in]
        n121 = Close File(refnum=w460, error in=w461) -> (error out=w445:errorcluster)  [unwired: 1 out]
      }
      frame "output" {
        n122 = Number To Decimal String(number=w483) -> (decimal integer string=w532:string)  [unwired: 1 in]
        n123 = Bundle By Name(cluster=w509, "Emergency Stop"=w535) -> (w545:T1)
        n124 = Delete From Array(array=w524, index=0 ("Index")) -> (deleted portion=w522:string, array with subset deleted=w521:string[])  [unwired: 1 in]
        n125 = Concatenate Strings(w531, "Prefix (output)", w532, w482, "Suffix (output)") -> (w534:string)
        n126 = VISA Write(VISA resource name=w500, write buffer=":PAGE:CHAN:MODE SWE;" ("write buffer (\"\")"), error in (no error)=w497) -> (VISA resource name out=w499:refnum<visa-resource-name>, error out=w498:errorcluster)  [unwired: 1 out]
        n127 = case shown="\"d\", Default" w522 {
          tunnel: [w546 w547] -> w520
          frame "s" {
            w546 = u16 0 items=["Single", "Double"] ("sweep mode")
          }
          frame "d", Default {
            w547 = u16 1 items=["Single", "Double"] ("sweep mode")
          }
        }
        n128 = Fract/Exp String To Number(string=w521) -> (number=w503:dbl[])  [unwired: 3 in, 1 out]
        n129 = String To Path(string=w534) -> (path=w530:path)
        n130 = Index Array(array=w503, index #1=0 ("Index")) -> (element #1=w519:dbl, element #2=w518:dbl, element #3=w517:dbl)  [unwired: 2 in]
        n131 = Delete From Array(array=w503, length=3 ("Length"), index=0 ("Index")) -> (array with subset deleted=w502:dbl[])  [unwired: 1 out]
        n132 = control-ref of="I vs Vd"() -> (w473:refnum<vi>)
        n133 = Bundle By Name(cluster=w511, "Gate Start"=w519, "Gate Stop"=w518, "Gate Step (linear only)"=w517, "Gate Compliance"=w528, "Range mode"=w495, "Range"=w494) -> (w544:T4)
        n134 = Index Array(array=w502, index #1=0 ("Index")) -> (element #1=w514:dbl, element #2=w513:dbl, element #3=w512:dbl)  [unwired: 2 in]
        n135 = call <vilib>:"compatOverwrite.vi"("overwrite (F)"=TRUE) -> ("overwrite?"=w487:T7)
        n136 = Bundle By Name(cluster=w510, "Drain Start"=w514, "Drain Stop"=w513, "Drain Step"=w512, "Drain Compliance"=w529, "Range mode"=w493, "Range"=w496) -> (w543:T5)
        n137 = call "4155C Output.vi"("VISA resource name in"=w499, "Gate"=w544, "Drain"=w543, "Timings"=w527, "error in (no error)"=w498, "SMU4"=w489, "sweep mode"=w520, "Panel controls"=w545) -> ("VD"=w480:dbl[], "Outparams"=w491:T8, "VISA Resource Name out"=w526:refnum<visa-resource-name>, "IS"=w479:dbl[], "ID"=w478:dbl[], "IG"=w477:dbl[], "error out"=w475:errorcluster, "SMU4"=w488:dbl[])  [unwired: 12 in]
        n138 = Unbundle By Name(w491) -> ("V2 Step"=w492:dbl, "V2 Start"=w490:dbl, "Number of points"=w472:i32)
        n139 = call "4155C Split array.vi"("Number of VAR2 steps"=w472, "Y2 data in"=w478, "X data in"=w480, "Y1 data in"=w479, "Y3 data in"=w477, "error in (no error)"=w475) -> ("Array of clusters"=w476:cluster{"Y data in":dbl[], "X data in":dbl[]}[], "error out"=w474:errorcluster)  [unwired: 1 in]
        n140 = local write "I vs Vd"(w476) -> ()
        n141 = call "4155C Config Chart Colours.vi"("Numeric"=w472, "XY Graph 2"=w473) -> ()  [unwired: 6 in]
        n142 = Open/Create/Replace File(file path (use dialog)=w530, error in=w474, operation (0:open)=w487) -> (refnum out=w540:refnum<file>, error out=w541:errorcluster)  [unwired: 3 in, 1 out]
        n143 = call "4155C Make Big 2d array.vi"("1D Var1"=w480, "1d IS"=w479, "1d ID"=w478, "1d IG"=w477, "1d SMU4"=w488, "SMU4"=w489, "VAR2 START"=w490, "Number of VAR2 steps"=w472, "VAR2 STEP"=w492, "VAR1 Name"="Vd", "Decimal places in header"=i8 1, "VAR2 Name"="Vg") -> ("Header array"=w536:string[], "Data array"=w537:dbl[][])  [unwired: 14 in]
        n144 = call "4155C Write array to file.vi"("Byte Stream File Refnum"=w540, "Header"=w536, "Data Array"=w537, "error in (no error)"=w541) -> ("dup refnum"=w538:refnum<file>, "error out"=w539:errorcluster)  [unwired: 1 in]
        n145 = Close File(refnum=w538, error in=w539) -> (error out=w525:errorcluster)  [unwired: 1 out]
      }
      frame "output-fpp" {
        n146 = Number To Decimal String(number=w554) -> (decimal integer string=w608:string)  [unwired: 1 in]
        n147 = Bundle By Name(cluster=w584, "Emergency Stop"=w611) -> (w621:T1)
        n148 = Delete From Array(array=w599, index=0 ("Index")) -> (deleted portion=w597:string, array with subset deleted=w596:string[])  [unwired: 1 in]
        n149 = VISA Write(VISA resource name=w575, write buffer=":PAGE:CHAN:MODE SWE;" ("write buffer (\"\")"), error in (no error)=w572) -> (VISA resource name out=w574:refnum<visa-resource-name>, error out=w573:errorcluster)  [unwired: 1 out]
        n150 = Concatenate Strings(w607, "-outputfpp-" ("Substring"), w608, w553, ".txt" ("Substring")) -> (w610:string)
        n151 = case shown="\"d\", Default" w597 {
          tunnel: [w622 w623] -> w595
          frame "s" {
            w622 = u16 0 items=["Single", "Double"] ("sweep mode")
          }
          frame "d", Default {
            w623 = u16 1 items=["Single", "Double"] ("sweep mode")
          }
        }
        n152 = Fract/Exp String To Number(string=w596) -> (number=w578:dbl[])  [unwired: 3 in, 1 out]
        n153 = String To Path(string=w610) -> (path=w606:path)
        n154 = Index Array(array=w578, index #1=0 ("Index")) -> (element #1=w594:dbl, element #2=w593:dbl, element #3=w592:dbl)  [unwired: 2 in]
        n155 = Delete From Array(array=w578, length=3 ("Length"), index=0 ("Index")) -> (array with subset deleted=w577:dbl[])  [unwired: 1 out]
        n156 = Bundle By Name(cluster=w586, "Gate Start"=w594, "Gate Stop"=w593, "Gate Step (linear only)"=w592, "Gate Compliance"=w604, "Range mode"=w570, "Range"=w569) -> (w620:T4)
        n157 = Index Array(array=w577, index #1=0 ("Index")) -> (element #1=w589:dbl, element #2=w588:dbl, element #3=w587:dbl)  [unwired: 2 in]
        n158 = call <vilib>:"compatOverwrite.vi"("overwrite (F)"=TRUE) -> ("overwrite?"=w558:T7)
        n159 = Bundle By Name(cluster=w585, "Drain Start"=w589, "Drain Stop"=w588, "Drain Step"=w587, "Drain Compliance"=w605, "Range mode"=w568, "Range"=w571) -> (w619:T5)
        n160 = call "4155C Output-FPP.vi"("VISA resource name in"=w574, "Gate"=w620, "Drain"=w619, "Timings"=w603, "error in (no error)"=w573, "sweep mode"=w595, "Panel controls"=w621) -> ("VD"=w563:dbl[], "Outparams"=w566:T8, "VISA Resource Name out"=w601:refnum<visa-resource-name>, "Vprobe2"=w562:dbl[], "ID"=w561:dbl[], "IG"=w560:dbl[], "Vprobe1"=w559:dbl[], "error out"=w602:errorcluster)  [unwired: 13 in]
        n161 = Unbundle By Name(w566) -> ("V2 Step"=w567:dbl, "V2 Start"=w565:dbl, "Number of points"=w564:i32)
        n162 = Open/Create/Replace File(file path (use dialog)=w606, error in=w602, operation (0:open)=w558) -> (refnum out=w616:refnum<file>, error out=w617:errorcluster)  [unwired: 3 in, 1 out]
        n163 = call "4155C Make Big 2d array FPP.vi"("1D Var1"=w563, "1d ID"=w561, "1d Vp2"=w562, "1d IG"=w560, "1d Vp1"=w559, "VAR2 START"=w565, "Number of VAR2 steps"=w564, "VAR2 STEP"=w567, "VAR1 Name"="Vd", "Decimal places in header"=i8 1, "VAR2 Name"="Vg") -> ("Header array"=w612:string[], "Data array"=w613:dbl[][])  [unwired: 15 in]
        n164 = call "4155C Write array to file.vi"("Byte Stream File Refnum"=w616, "Header"=w612, "Data Array"=w613, "error in (no error)"=w617) -> ("dup refnum"=w614:refnum<file>, "error out"=w615:errorcluster)  [unwired: 1 in]
        n165 = Close File(refnum=w614, error in=w615) -> (error out=w600:errorcluster)  [unwired: 1 out]
      }
      frame "itime" {
        n166 = Delete From Array(array=w642, index=0 ("Index")) -> (deleted portion=w643:string)  [unwired: 1 in, 1 out]
        n167 = case shown="\"l\"" w643 {
          tunnel: w641 -> [w647 w649 w652]
          tunnel: [w646 w648 w651] -> w634
          frame "s" {
            w645 = u32 0 items=["short  ", "medium  ", "long  "] ("integration time 2")
            n168 = Bundle By Name(cluster=w647, "integration time"=w645) -> (w646:T6)
          }
          frame "m", Default {
            w650 = u32 1 items=["short  ", "medium  ", "long  "] ("integration time 2")
            n169 = Bundle By Name(cluster=w649, "integration time"=w650) -> (w648:T6)
          }
          frame "l" {
            w653 = u32 2 items=["short  ", "medium  ", "long  "] ("integration time 2")
            n170 = Bundle By Name(cluster=w652, "integration time"=w653) -> (w651:T6)
          }
        }
      }
      frame "pulsed" {
        n171 = Delete From Array(array=w673, index=0 ("Index")) -> (deleted portion=w674:string, array with subset deleted=w661:string[])  [unwired: 1 in]
        n172 = case shown="\"on\", Default" w674 {
          tunnel: w672 -> [w684 w687]
          tunnel: [w683 w686] -> w665
          tunnel: w661 -> [w681 _]
          frame "on", Default {
            w682 = u16 1 items=["Continuous", "Pulsed"] ("sweep method")
            n173 = Fract/Exp String To Number(string=w681) -> (number=w679:dbl[])  [unwired: 3 in, 1 out]
            n174 = Index Array(array=w679, index #1=0 ("Index")) -> (element #1=w678:dbl, element #2=w677:dbl, element #3=w676:dbl)  [unwired: 2 in]
            n175 = Bundle By Name(cluster=w684, "sweep method"=w682, "Pulse period"=w678, "Base voltage"=w677, "Pulse width"=w676) -> (w683:T6)
          }
          frame "off" {
            w685 = u16 0 items=["Continuous", "Pulsed"] ("sweep method")
            n176 = Bundle By Name(cluster=w687, "sweep method"=w685) -> (w686:T6)
          }
        }
      }
      frame "gaterangemode" {
        n177 = Delete From Array(array=w705, index=0 ("Index")) -> (deleted portion=w706:string)  [unwired: 1 in, 1 out]
        n178 = case shown="\"f\"" w706 {
          tunnel: [w708 w709 w710] -> w695
          frame "a", Default {
            w708 = u16 0 items=["Auto", "Limited", "Fixed"] ("Gate Range\nmode 2")
          }
          frame "f" {
            w709 = u16 2 items=["Auto", "Limited", "Fixed"] ("Gate Range\nmode 2")
          }
          frame "l" {
            w710 = u16 1 items=["Auto", "Limited", "Fixed"] ("Gate Range\nmode 2")
          }
        }
      }
      frame "gaterange" {
        (unwired) u8 11 items=["10fA  ", "100fA  ", "1nA  ", "10nA", "100nA", "1uA", "10uA", "100uA", "1mA", "10mA", "100mA", "1A"] ("Gate Range 2")
        n179 = Delete From Array(array=w735, index=0 ("Index")) -> (deleted portion=w725:string)  [unwired: 1 in, 1 out]
        n180 = Scan Value(string=w725, format string="") -> (value=w723:dbl)  [unwired: 1 in, 1 out]
        n181 = Logarithm Base 10(1:w723) -> (0:w722:dbl)
        n182 = Round To Nearest(number=w722) -> (nearest integer value=w721:dbl)
        n183 = Add(x=w721, y=11.0) -> (x+y=w719:dbl)
        n184 = To Unsigned Byte Integer(number=w719) -> (unsigned 8bit integer=w718:u8)
      }
      frame "drainrange" {
        (unwired) u8 11 items=["10fA  ", "100fA  ", "1nA  ", "10nA", "100nA", "1uA", "10uA", "100uA", "1mA", "10mA", "100mA", "1A"] ("Gate Range 2")
        n185 = Delete From Array(array=w761, index=0 ("Index")) -> (deleted portion=w752:string)  [unwired: 1 in, 1 out]
        n186 = Scan Value(string=w752, format string="") -> (value=w750:dbl)  [unwired: 1 in, 1 out]
        n187 = Logarithm Base 10(1:w750) -> (0:w749:dbl)
        n188 = Round To Nearest(number=w749) -> (nearest integer value=w748:dbl)
        n189 = Add(x=w748, y=11.0) -> (x+y=w746:dbl)
        n190 = To Unsigned Byte Integer(number=w746) -> (unsigned 8bit integer=w745:u8)
      }
      frame "drainrangemode" {
        n191 = Delete From Array(array=w780, index=0 ("Index")) -> (deleted portion=w781:string)  [unwired: 1 in, 1 out]
        n192 = case shown="\"f\"" w781 {
          tunnel: [w783 w784 w785] -> w770
          frame "a", Default {
            w783 = u16 0 items=["Auto", "Limited", "Fixed"] ("Gate Range\nmode 2")
          }
          frame "f" {
            w784 = u16 2 items=["Auto", "Limited", "Fixed"] ("Gate Range\nmode 2")
          }
          frame "l" {
            w785 = u16 1 items=["Auto", "Limited", "Fixed"] ("Gate Range\nmode 2")
          }
        }
      }
      frame "Error", Default {
      }
      frame "logfile" {
        n193 = Number To Decimal String(number=w810) -> (decimal integer string=w845:string)  [unwired: 1 in]
        n194 = Concatenate Strings(w844, "logfile" ("Substring"), w845, w808, ".txt" ("Substring")) -> (w842:string)
        n195 = String To Path(string=w842) -> (path=w815:path)
        n196 = Unbundle(w841) -> ("integration time"=w840:u32, "Short/Long integration time"=w839:dbl, "hold time (sec)"=w838:dbl, "delay time (sec)"=w837:dbl, "Step Time (0 disables)"=w836:dbl, "sweep method"=w835:u16, "Pulse period"=w834:dbl, "Base voltage"=w833:dbl, "Pulse width"=w832:dbl)
        n197 = Build Array(w840, w839, w838, w837, w836, w835, w834, w833, w832, w826, w827, w828, w829, w830, w831) -> (w819:dbl[])
        n198 = Insert Into Array(array=dbl[][] [] ("Input Array"), new element=w819) -> (w818:dbl[][])  [unwired: 2 in]
        n199 = call <vilib>:"compatOverwrite.vi"("overwrite (F)"=TRUE) -> ("overwrite?"=w813:T7)
        n200 = Open/Create/Replace File(file path (use dialog)=w815, error in=w817, operation (0:open)=w813) -> (refnum out=w823:refnum<file>, error out=w822:errorcluster)  [unwired: 3 in, 1 out]
        n201 = call "4155C Write array to file.vi"("Byte Stream File Refnum"=w823, "Header"=string[] ["Int Time", "Short/Long Itime", "Hold time", "Delay time", "Step time", "Sweep method", "Pulse period", "Base Voltage", "Pulse width", "Drain compliance", "Gate compliance", "Gate range mode", "Gate range", "S/D range mode", "S/D range"], "Data Array"=w818, "error in (no error)"=w822) -> ("dup refnum"=w825:refnum<file>, "error out"=w824:errorcluster)  [unwired: 1 in]
        n202 = Close File(refnum=w825, error in=w824) -> (error out=w816:errorcluster)  [unwired: 1 out]
      }
      frame "sample" {
        n203 = Number To Decimal String(number=w854) -> (decimal integer string=w902:string)  [unwired: 1 in]
        n204 = Fract/Exp String To Number(string=w899) -> (number=w860:dbl[])  [unwired: 3 in, 1 out]
        n205 = Concatenate Strings(w877, "-sample-" ("Substring"), w902, w852, ".txt" ("Substring")) -> (w900:string)
        n206 = String To Path(string=w900) -> (path=w881:path)
        n207 = Index Array(array=w860, index=0 ("Index")) -> (element=w897:dbl)
        n208 = Index Array(array=w860, index=2 ("Index")) -> (element=w893:dbl)
        n209 = Index Array(array=w860, index=3 ("Index")) -> (element=w862:dbl)
        n210 = Index Array(array=w860, index=4 ("Index")) -> (element=w859:dbl)
        n211 = call "4155C Config Sampling Measurements.vi"("Sampling interval"=w859, "Sample time"=w862, "Display on/off"=TRUE, "Timings"=w868, "Num Points"=w893, "error in (no error)"=w904, "Drain Compliance"=w903, "Gate Compliance"=w878, "VISA session"=w905) -> ("error out"=w906:errorcluster, "dup VISA resource name"=w907:refnum<visa-resource-name>)  [unwired: 1 in]
        n212 = Index Array(array=w860, index=1 ("Index")) -> (element=w894:dbl)
        n213 = call "4155C Take Sample.vi"("Emergency Stop"=w874, "error in (no error)"=w906, "Vd"=w894, "Vg"=w897, "VISA resource name in"=w907) -> ("error out"=w872:errorcluster, "Id"=w909:dbl[], "Ig"=w883:dbl[], "VISA Resource Name out"=w870:refnum<visa-resource-name>, "Is"=w908:dbl[], "Time"=w887:dbl[])  [unwired: 1 in]
        n214 = Insert Into Array(array=dbl[][] [] ("Input Array"), new element=w887) -> (w886:dbl[][])  [unwired: 2 in]
        n215 = Insert Into Array(array=w886, new element=w883) -> (w885:dbl[][])  [unwired: 2 in]
        n216 = Insert Into Array(array=w885, new element=w909) -> (w884:dbl[][])  [unwired: 2 in]
        n217 = VISA Write(VISA resource name=w870, write buffer=":DISP ON" ("write buffer (\"\")"), error in (no error)=w872) -> (VISA resource name out=w869:refnum<visa-resource-name>, error out=w871:errorcluster)  [unwired: 1 out]
        n218 = Insert Into Array(array=w884, new element=w908) -> (w876:dbl[][])  [unwired: 2 in]
        n219 = Transpose 2D Array(2D array=w876) -> (transposed array=w875:dbl[][])
        n220 = call <vilib>:"compatOverwrite.vi"("overwrite (F)"=TRUE) -> ("overwrite?"=w857:T7)
        n221 = Open/Create/Replace File(file path (use dialog)=w881, error in=w871, operation (0:open)=w857) -> (refnum out=w890:refnum<file>, error out=w889:errorcluster)  [unwired: 3 in, 1 out]
        n222 = call "4155C Write array to file.vi"("Byte Stream File Refnum"=w890, "Header"=string[] ["Time /s", "Ig /A", "Id /A", "Is /A"], "Data Array"=w875, "error in (no error)"=w889) -> ("dup refnum"=w892:refnum<file>, "error out"=w891:errorcluster)  [unwired: 1 in]
        n223 = Close File(refnum=w892, error in=w891) -> (error out=w879:errorcluster)  [unwired: 1 out]
      }
      frame "samplei" {
        n224 = Number To Decimal String(number=w916) -> (decimal integer string=w968:string)  [unwired: 1 in]
        n225 = Fract/Exp String To Number(string=w965) -> (number=w932:dbl[])  [unwired: 3 in, 1 out]
        n226 = Concatenate Strings(w947, "-samplei-" ("Substring"), w968, w915, ".txt" ("Substring")) -> (w966:string)
        n227 = String To Path(string=w966) -> (path=w950:path)
        n228 = Index Array(array=w932, index=4 ("Index")) -> (element=w926:dbl)
        n229 = Index Array(array=w932, index=3 ("Index")) -> (element=w927:dbl)
        n230 = Index Array(array=w932, index=1 ("Index")) -> (element=w929:dbl)
        n231 = Index Array(array=w932, index=0 ("Index")) -> (element=w930:dbl)
        n232 = Index Array(array=w932, index=2 ("Index")) -> (element=w928:dbl)
        n233 = call "4155C Config SamplingI Measurements.vi"("Sample time"=w928, "Display on/off"=TRUE, "Timings"=w939, "Num Points"=w929, "error in (no error)"=w970, "Sampling interval"=w927, "VISA session"=w971) -> ("error out"=w972:errorcluster, "dup VISA resource name"=w973:refnum<visa-resource-name>)  [unwired: 3 in]
        n234 = call "4155C Take SampleI.vi"("Emergency Stop"=w944, "error in (no error)"=w972, "Idg 2"=w930, "Vdg compliance 2"=w926, "VISA resource name in"=w973) -> ("error out"=w942:errorcluster, "Idg"=w975:dbl[], "Vdg"=w952:dbl[], "VISA Resource Name out"=w940:refnum<visa-resource-name>, "Is"=w974:dbl[], "Time"=w956:dbl[])  [unwired: 1 in]
        n235 = Insert Into Array(array=dbl[][] [] ("Input Array"), new element=w956) -> (w955:dbl[][])  [unwired: 2 in]
        n236 = Insert Into Array(array=w955, new element=w952) -> (w954:dbl[][])  [unwired: 2 in]
        n237 = Insert Into Array(array=w954, new element=w975) -> (w953:dbl[][])  [unwired: 2 in]
        n238 = VISA Write(VISA resource name=w940, write buffer=":DISP ON" ("write buffer (\"\")"), error in (no error)=w942) -> (VISA resource name out=w925:refnum<visa-resource-name>, error out=w941:errorcluster)  [unwired: 1 out]
        n239 = Insert Into Array(array=w953, new element=w974) -> (w946:dbl[][])  [unwired: 2 in]
        n240 = Transpose 2D Array(2D array=w946) -> (transposed array=w945:dbl[][])
        n241 = call <vilib>:"compatOverwrite.vi"("overwrite (F)"=TRUE) -> ("overwrite?"=w920:T7)
        n242 = Open/Create/Replace File(file path (use dialog)=w950, error in=w941, operation (0:open)=w920) -> (refnum out=w959:refnum<file>, error out=w958:errorcluster)  [unwired: 3 in, 1 out]
        n243 = call "4155C Write array to file.vi"("Byte Stream File Refnum"=w959, "Header"=string[] ["Time /s", "Vdg /V", "Idg /A", "Is /A"], "Data Array"=w945, "error in (no error)"=w958) -> ("dup refnum"=w961:refnum<file>, "error out"=w960:errorcluster)  [unwired: 1 in]
        n244 = Close File(refnum=w961, error in=w960) -> (error out=w923:errorcluster)  [unwired: 1 out]
        n245 = VISA Write(VISA resource name=w925, write buffer=";:PAGE:SCON:STAN OFF;:PAGE:CHAN:VSU2:DIS;" ("write buffer (\"\")"), error in (no error)=w923) -> (VISA resource name out=w921:refnum<visa-resource-name>, error out=w922:errorcluster)  [unwired: 1 out]
      }
      frame "#" {
        n246 = VISA Write(VISA resource name=w987, write buffer=":DISP ON" ("write buffer (\"\")"), error in (no error)=w986) -> (VISA resource name out=w985:refnum<visa-resource-name>, error out=w984:errorcluster)  [unwired: 1 out]
      }
      frame "stressV" {
        n247 = Number To Decimal String(number=w1002) -> (decimal integer string=w1043:string)  [unwired: 1 in]
        n248 = Fract/Exp String To Number(string=w1040) -> (number=w1013:dbl[])  [unwired: 3 in, 1 out]
        n249 = Concatenate Strings(w1027, "-stressV-" ("Substring"), w1043, w1001, ".txt" ("Substring")) -> (w1041:string)
        n250 = String To Path(string=w1041) -> (path=w1031:path)
        n251 = Index Array(array=w1013, index=3 ("Index")) -> (element=w1010:dbl)
        n252 = Index Array(array=w1013, index=1 ("Index")) -> (element=w1008:dbl)
        n253 = Index Array(array=w1013, index=0 ("Index")) -> (element=w1007:dbl)
        n254 = Index Array(array=w1013, index=4 ("Index")) -> (element=w1012:dbl)
        n255 = Index Array(array=w1013, index=2 ("Index")) -> (element=w1009:dbl)
        n256 = call "4155C Config V Stress.vi"("VISA session"=w1046, "ID compliance"=w1010, "VD"=w1008, "VG"=w1007, "IG compliance"=w1009, "error in (no error)"=w1045, "Display on/off"=TRUE) -> ("dup VISA resource name"=w1048:refnum<visa-resource-name>, "error out"=w1047:errorcluster)
        n257 = call "4155C Apply Stress.vi"("error in (no error)"=w1047, "Duration"=w1012, "Emergency Stop"=w1026, "VISA resource name in"=w1048) -> ("error out"=w1024:errorcluster, "VISA Resource Name out"=w1022:refnum<visa-resource-name>)
        n258 = VISA Write(VISA resource name=w1022, write buffer=":DISP ON" ("write buffer (\"\")"), error in (no error)=w1024) -> (VISA resource name out=w1021:refnum<visa-resource-name>, error out=w1023:errorcluster)  [unwired: 1 out]
        n259 = call <vilib>:"compatOverwrite.vi"("overwrite (F)"=TRUE) -> ("overwrite?"=w1006:T7)
        n260 = Open/Create/Replace File(file path (use dialog)=w1031, error in=w1023, operation (0:open)=w1006) -> (refnum out=w1034:refnum<file>, error out=w1033:errorcluster)  [unwired: 3 in, 1 out]
        n261 = call "4155C Write array to file.vi"("Byte Stream File Refnum"=w1034, "Header"=string[] ["V stress completed successfully", ""], "error in (no error)"=w1033) -> ("dup refnum"=w1036:refnum<file>, "error out"=w1035:errorcluster)  [unwired: 2 in]
        n262 = Close File(refnum=w1036, error in=w1035) -> (error out=w1029:errorcluster)  [unwired: 1 out]
      }
      frame "stressI" {
        n263 = Number To Decimal String(number=w1055) -> (decimal integer string=w1092:string)  [unwired: 1 in]
        n264 = Fract/Exp String To Number(string=w1089) -> (number=w1064:dbl[])  [unwired: 3 in, 1 out]
        n265 = Concatenate Strings(w1076, "-stressI-" ("Substring"), w1092, w1054, ".txt" ("Substring")) -> (w1090:string)
        n266 = String To Path(string=w1090) -> (path=w1080:path)
        n267 = Index Array(array=w1064, index=1 ("Index")) -> (element=w1060:dbl)
        n268 = Index Array(array=w1064, index=0 ("Index")) -> (element=w1061:dbl)
        n269 = call "4155C Config I Stress.vi"("VISA session"=w1095, "IDG"=w1061, "VDG compliance"=w1060, "error in (no error)"=w1094, "Display on/off"=TRUE) -> ("dup VISA resource name"=w1097:refnum<visa-resource-name>, "error out"=w1096:errorcluster)
        n270 = Index Array(array=w1064, index=2 ("Index")) -> (element=w1062:dbl)
        n271 = call "4155C Apply Stress.vi"("error in (no error)"=w1096, "Duration"=w1062, "Emergency Stop"=w1075, "VISA resource name in"=w1097) -> ("error out"=w1073:errorcluster, "VISA Resource Name out"=w1071:refnum<visa-resource-name>)
        n272 = VISA Write(VISA resource name=w1071, write buffer=":DISP ON" ("write buffer (\"\")"), error in (no error)=w1073) -> (VISA resource name out=w1070:refnum<visa-resource-name>, error out=w1072:errorcluster)  [unwired: 1 out]
        n273 = call <vilib>:"compatOverwrite.vi"("overwrite (F)"=TRUE) -> ("overwrite?"=w1059:T7)
        n274 = Open/Create/Replace File(file path (use dialog)=w1080, error in=w1072, operation (0:open)=w1059) -> (refnum out=w1083:refnum<file>, error out=w1082:errorcluster)  [unwired: 3 in, 1 out]
        n275 = call "4155C Write array to file.vi"("Byte Stream File Refnum"=w1083, "Header"=string[] ["I stress completed successfully", ""], "error in (no error)"=w1082) -> ("dup refnum"=w1085:refnum<file>, "error out"=w1084:errorcluster)  [unwired: 2 in]
        n276 = Close File(refnum=w1085, error in=w1084) -> (error out=w1078:errorcluster)  [unwired: 1 out]
      }
      frame "vsu2pulse" {
        n277 = Number To Decimal String(number=w1104) -> (decimal integer string=w1139:string)  [unwired: 1 in]
        n278 = Fract/Exp String To Number(string=w1136) -> (number=w1112:dbl[])  [unwired: 3 in, 1 out]
        n279 = Concatenate Strings(w1124, "-vsu2-" ("Substring"), w1139, w1103, ".txt" ("Substring")) -> (w1137:string)
        n280 = String To Path(string=w1137) -> (path=w1128:path)
        n281 = Index Array(array=w1112, index=1 ("Index")) -> (element=w1111:dbl)
        n282 = Index Array(array=w1112, index=0 ("Index")) -> (element=w1109:dbl)
        n283 = call "4155C Config VSU2 Stress.vi"("error in (no error)"=w1141, "VSU2"=w1109, "Display on/off"=TRUE, "VISA session"=w1142) -> ("error out"=w1143:errorcluster, "dup VISA resource name"=w1144:refnum<visa-resource-name>)
        n284 = call "4155C Apply Stress.vi"("error in (no error)"=w1143, "Duration"=w1111, "Emergency Stop"=w1123, "VISA resource name in"=w1144) -> ("error out"=w1121:errorcluster, "VISA Resource Name out"=w1119:refnum<visa-resource-name>)
        n285 = VISA Write(VISA resource name=w1119, write buffer=":DISP ON" ("write buffer (\"\")"), error in (no error)=w1121) -> (VISA resource name out=w1118:refnum<visa-resource-name>, error out=w1120:errorcluster)  [unwired: 1 out]
        n286 = call <vilib>:"compatOverwrite.vi"("overwrite (F)"=TRUE) -> ("overwrite?"=w1108:T7)
        n287 = Open/Create/Replace File(file path (use dialog)=w1128, error in=w1120, operation (0:open)=w1108) -> (refnum out=w1131:refnum<file>, error out=w1130:errorcluster)  [unwired: 3 in, 1 out]
        n288 = call "4155C Write array to file.vi"("Byte Stream File Refnum"=w1131, "Header"=string[] ["VSU2 pulse completed successfully", ""], "error in (no error)"=w1130) -> ("dup refnum"=w1133:refnum<file>, "error out"=w1132:errorcluster)  [unwired: 2 in]
        n289 = Close File(refnum=w1133, error in=w1132) -> (error out=w1126:errorcluster)  [unwired: 1 out]
      }
      frame "sample-fpp" {
        w1162 = string[] ["Time /s", "Id VgVd /A", "Ig VgVd /A", "Vp1 VgVd /V", "Vp2 VgVd /V"] ("Header")
        w1166 = "%d" ("format string")
        n290 = Number To Decimal String(number=w1151) -> (decimal integer string=w1214:string)  [unwired: 1 in]
        n291 = Fract/Exp String To Number(string=w1211) -> (number=w1199:dbl[])  [unwired: 3 in, 1 out]
        n292 = Concatenate Strings(w1205, "-samplefpp-" ("Substring"), w1214, w1150, ".txt" ("Substring")) -> (w1212:string)
        n293 = String To Path(string=w1212) -> (path=w1174:path)
        n294 = Index Array(array=w1199, index=0 ("Index")) -> (element=w1160:dbl)
        n295 = Index Array(array=w1199, index=1 ("Index")) -> (element=w1159:dbl)
        n296 = Index Array(array=w1199, index=2 ("Index")) -> (element=w1207:dbl)
        n297 = Index Array(array=w1199, index=3 ("Index")) -> (element=w1197:dbl)
        n298 = call "4155C Config Sampling Measurements FPP.vi"("VISA session"=w1217, "Num Points"=w1207, "Vg"=w1160, "Display on/off"=TRUE, "Gate Compliance"=w1206, "Drain Compliance"=w1215, "Standby"="Standby", "error in (no error)"=w1216, "Timings"=w1204, "Vd"=w1159, "Sample time"=w1197) -> ("dup VISA resource name"=w1176:refnum<visa-resource-name>, "error out"=w1175:errorcluster)  [unwired: 3 in]
        n299 = Number To Decimal String(number=w1160) -> (decimal integer string=w1186:string)  [unwired: 1 in]
        n300 = call "4155C Take Sample FPP.vi"("VISA resource name in"=w1176, "error in (no error)"=w1175, "Emergency Stop"=w1177) -> ("Time"=w1181:dbl[], "Vp1"=w1191:dbl[], "VISA Resource Name out"=w1157:refnum<visa-resource-name>, "Ig"=w1179:dbl[], "Id"=w1180:dbl[], "Vp2"=w1189:dbl[], "error out"=w1178:errorcluster)  [unwired: 10 in]
        n301 = Insert Into Array(array=dbl[][] [] ("Input Array"), new element=w1181) -> (w1195:dbl[][])  [unwired: 2 in]
        n302 = Number To Decimal String(number=w1159) -> (decimal integer string=w1184:string)  [unwired: 1 in]
        n303 = Insert Into Array(array=w1195, new element=w1180) -> (w1194:dbl[][])  [unwired: 2 in]
        n304 = Concatenate Strings("(Vg = " ("Substring"), w1186, "V, Vd = " ("Substring"), w1184, "V)" ("Substring")) -> (w1182:string)
        n305 = Insert Into Array(array=w1194, new element=w1179) -> (w1193:dbl[][])  [unwired: 2 in]
        n306 = Insert Into Array(array=w1193, new element=w1191) -> (w1190:dbl[][])  [unwired: 2 in]
        n307 = Insert Into Array(array=w1190, new element=w1189) -> (w1158:dbl[][])  [unwired: 2 in]
        n308 = call <vilib>:"compatOverwrite.vi"("overwrite (F)"=TRUE) -> ("overwrite?"=w1155:T7)
        n309 = Open/Create/Replace File(file path (use dialog)=w1174, error in=w1178, operation (0:open)=w1155) -> (refnum out=w1171:refnum<file>, error out=w1172:errorcluster)  [unwired: 3 in, 1 out]
        n310 = Array To Spreadsheet String(array=w1162, 3:w1166) -> (spreadsheet string=w1168:string)  [unwired: 1 in]
        n311 = Transpose 2D Array(2D array=w1158) -> (transposed array=w1188:dbl[][])
        n312 = Search and Replace String(replace all?=TRUE ("replace all? (F)"), input string=w1168, search string="VgVd", replace string=w1182) -> (result string=w1164:string)  [unwired: 4 in, 3 out]
        n313 = Spreadsheet String To Array(format string=w1166, spreadsheet string=w1164, array type (2D Dbl)=w1162) -> (array=w1163:string[])  [unwired: 1 in]
        n314 = call "4155C Write array to file.vi"("Byte Stream File Refnum"=w1171, "Header"=w1163, "Data Array"=w1188, "error in (no error)"=w1172) -> ("dup refnum"=w1169:refnum<file>, "error out"=w1170:errorcluster)  [unwired: 1 in]
        n315 = Close File(refnum=w1169, error in=w1170) -> (error out=w1156:errorcluster)  [unwired: 1 out]
      }
      frame "resample-fpp" {
        w1237 = string[] ["Time /s", "Id VgVd /A", "Ig VgVd /A", "Vp1 VgVd /V", "Vp2 VgVd /V"] ("Header")
        w1241 = "%d" ("format string")
        n316 = Number To Decimal String(number=w1223) -> (decimal integer string=w1281:string)  [unwired: 1 in]
        n317 = Fract/Exp String To Number(string=w1278) -> (number=w1230:dbl[])  [unwired: 3 in, 1 out]
        n318 = Concatenate Strings(w1274, "-resamplefpp-" ("Substring"), w1281, w1224, ".txt" ("Substring")) -> (w1279:string)
        n319 = String To Path(string=w1279) -> (path=w1249:path)
        n320 = Index Array(array=w1230, index=0 ("Index")) -> (element=w1236:dbl)
        n321 = Index Array(array=w1230, index=1 ("Index")) -> (element=w1235:dbl)
        n322 = Number To Decimal String(number=w1236) -> (decimal integer string=w1259:string)  [unwired: 1 in]
        n323 = call "4155C Take Sample FPP.vi"("VISA resource name in"=w1232, "error in (no error)"=w1231, "Emergency Stop"=w1250) -> ("Time"=w1254:dbl[], "Vp1"=w1264:dbl[], "VISA Resource Name out"=w1234:refnum<visa-resource-name>, "Ig"=w1252:dbl[], "Id"=w1253:dbl[], "Vp2"=w1262:dbl[], "error out"=w1251:errorcluster)  [unwired: 10 in]
        n324 = Insert Into Array(array=dbl[][] [] ("Input Array"), new element=w1254) -> (w1268:dbl[][])  [unwired: 2 in]
        n325 = Number To Decimal String(number=w1235) -> (decimal integer string=w1257:string)  [unwired: 1 in]
        n326 = Insert Into Array(array=w1268, new element=w1253) -> (w1267:dbl[][])  [unwired: 2 in]
        n327 = Concatenate Strings("(Vg = " ("Substring"), w1259, "V, Vd = " ("Substring"), w1257, "V)" ("Substring")) -> (w1255:string)
        n328 = Insert Into Array(array=w1267, new element=w1252) -> (w1266:dbl[][])  [unwired: 2 in]
        n329 = Insert Into Array(array=w1266, new element=w1264) -> (w1263:dbl[][])  [unwired: 2 in]
        n330 = Insert Into Array(array=w1263, new element=w1262) -> (w1229:dbl[][])  [unwired: 2 in]
        n331 = call <vilib>:"compatOverwrite.vi"("overwrite (F)"=TRUE) -> ("overwrite?"=w1228:T7)
        n332 = Open/Create/Replace File(file path (use dialog)=w1249, error in=w1251, operation (0:open)=w1228) -> (refnum out=w1246:refnum<file>, error out=w1247:errorcluster)  [unwired: 3 in, 1 out]
        n333 = Array To Spreadsheet String(array=w1237, 3:w1241) -> (spreadsheet string=w1243:string)  [unwired: 1 in]
        n334 = Transpose 2D Array(2D array=w1229) -> (transposed array=w1261:dbl[][])
        n335 = Search and Replace String(replace all?=TRUE ("replace all? (F)"), input string=w1243, search string="VgVd", replace string=w1255) -> (result string=w1239:string)  [unwired: 4 in, 3 out]
        n336 = Spreadsheet String To Array(format string=w1241, spreadsheet string=w1239, array type (2D Dbl)=w1237) -> (array=w1238:string[])  [unwired: 1 in]
        n337 = call "4155C Write array to file.vi"("Byte Stream File Refnum"=w1246, "Header"=w1238, "Data Array"=w1261, "error in (no error)"=w1247) -> ("dup refnum"=w1244:refnum<file>, "error out"=w1245:errorcluster)  [unwired: 1 in]
        n338 = Close File(refnum=w1244, error in=w1245) -> (error out=w1233:errorcluster)  [unwired: 1 out]
      }
      frame "serial" {
        n339 = local read "Enable Termination\nChar (T)"() -> (w1296:bool)
        n340 = local read "Termination char\n(0xA = '\\n' = LF)\n(0xD = '\\r' = CR)"() -> (w1295:u8)
        n341 = Index Array(array=w1303, index=0 ("Index")) -> (element=w1302:string)
        n342 = local read "parity"() -> (w1286:u16)
        n343 = local read "Delay before read (ms)"() -> (w1297:u32)
        n344 = local read "byte count"() -> (w1294:u32)
        n345 = local read "Timeout (ms)"() -> (w1293:u32)
        n346 = local read "VISA resource name"() -> (w1290:refnum<visa-resource-name>)
        n347 = local read "baud rate"() -> (w1289:u32)
        n348 = local read "Serial End Mode for Reads"() -> (w1288:u16)
        n349 = local read "data bits"() -> (w1287:u16)
        n350 = local read "stop bits"() -> (w1292:u16)
        n351 = local read "flow control"() -> (w1291:u16)
        n352 = call "Serial write and read v0.5.vi"("Delay before read (ms)"=w1297, "Termination char\n(0xA = '\\n' = LF)\n(0xD = '\\r' = CR)"=w1295, "Enable Termination\nChar (T)"=w1296, "parity"=w1286, "stop bits"=w1292, "string to write"=w1302, "flow control"=w1291, "byte count"=w1294, "Serial Settings:Serial End Mode for Reads"=w1288, "Timeout (ms)"=w1293, "error in (no error)"=w1308, "VISA resource name"=w1290, "baud rate"=w1289, "data bits"=w1287) -> ("Serial port output"=w1298:string, "error out"=w1307:errorcluster)
        n353 = Build Array (concatenate)(w1298, w1299) -> (w1300:string[])
      }
      frame "pump" {
        # "Check if hard stop is pressed."
        # "Check if halt is pressed."
        # "Check if pump is idle. Else halt."
        n354 = local read "Hard stop pump"() -> (w1327:bool)
        n355 = local read "Halt pump"() -> (w1330:bool)
        n356 = local read "Enable Termination\nChar (T)"() -> (w1348:bool)
        n357 = local read "Termination char\n(0xA = '\\n' = LF)\n(0xD = '\\r' = CR)"() -> (w1347:u8)
        n358 = Index Array(array=w1352, index=0 ("Index")) -> (element=w1324:string)
        n359 = case shown="\"Initialization\"" w1321 {
          tunnel: w1324 -> [w1366 _ w1368 w1369 w1370 w1371 _ _ w1374 w1375 _]
          tunnel: [w1366 "/1H" w1368 w1369 w1370 w1371 "/1H" "/1H" w1374 w1375 "/1H"] -> w1323
          frame "No error", Default {
          }
          frame "Initialization" {
          }
          frame "Invalid command" {
          }
          frame "Invalid operand" {
          }
          frame "Device not initialized" {
          }
          frame "Internal failure" {
          }
          frame "Plunger overload" {
          }
          frame "Valve overload" {
          }
          frame "Plunger move not allowed" {
          }
          frame "A/D converter failure" {
          }
          frame "Command overflow" {
          }
        }
        n360 = case shown="True" w1330 {
          tunnel: [w1380 "/1H"] -> w1329
          tunnel: w1323 -> [w1380 _]
          frame False {
          }
          frame True {
            n361 = local write "Halt pump"(FALSE) -> ()
          }
        }
        n362 = case shown="True" w1327 {
          tunnel: [w1377 "/1T"] -> w1328
          tunnel: w1329 -> [w1377 _]
          frame False {
          }
          frame True {
            n363 = local write "Hard stop pump"(FALSE) -> ()
          }
        }
        n364 = local read "Serial End Mode for Reads"() -> (w1340:u16)
        n365 = local read "flow control"() -> (w1343:u16)
        n366 = local read "stop bits"() -> (w1344:u16)
        n367 = local read "parity"() -> (w1338:u16)
        n368 = local read "Delay before read (ms)"() -> (w1349:u32)
        n369 = local read "byte count"() -> (w1346:u32)
        n370 = local read "Timeout (ms)"() -> (w1345:u32)
        n371 = local read "VISA resource name"() -> (w1342:refnum<visa-resource-name>)
        n372 = local read "baud rate"() -> (w1341:u32)
        n373 = local read "data bits"() -> (w1339:u16)
        n374 = call "SPM Pump v0.3.vi"("Termination char\n(0xA = '\\n' = LF)\n(0xD = '\\r' = CR)"=w1347, "Enable Termination\nChar (T)"=w1348, "Timeout (ms)"=w1345, "Serial Settings:Serial End Mode for Reads"=w1340, "byte count"=w1346, "Delay before read (ms)"=w1349, "Time <input>"=w1320, "error in (no error)"=w1357, "Serial port input"=w1328, "VISA resource name"=w1342, "parity"=w1338, "baud rate"=w1341, "stop bits"=w1344, "data bits"=w1339, "flow control"=w1343) -> ("Pump status"=w1322:string, "Valve position"=w1326:i32, "Absolute plunger position"=w1325:i32, "Serial port output"=w1319:string, "error out"=w1356:errorcluster)  [unwired: 4 in, 4 out]
        n375 = Build Array (concatenate)(w1331, w1326) -> (w1332:i32[])
        n376 = Build Array (concatenate)(w1335, w1325) -> (w1336:i32[])
        n377 = call "4155C Split array.vi"("X data in"=w1334, "Y1 data in"=w1332) -> ("Array of clusters"=w1333:cluster{"Y data in":dbl[], "X data in":dbl[]}[])  [unwired: 5 in, 1 out]
        n378 = local write "Valve position vs time"(w1333) -> ()
        n379 = call "4155C Split array.vi"("X data in"=w1334, "Y1 data in"=w1336) -> ("Array of clusters"=w1337:cluster{"Y data in":dbl[], "X data in":dbl[]}[])  [unwired: 5 in, 1 out]
        n380 = local write "Absolute plunger position vs time"(w1337) -> ()
        n381 = Build Array (concatenate)(w1318, w1319) -> (w1350:string[])
      }
    }
    n382 = Build Array(w88, w87, w81, w55) -> (w86:dbl[][])
    n383 = Concatenate Strings(w59, "-Serial port output", ".txt" ("Suffix")) -> (w63:string)
    n384 = Build Array("Time /s" ("element"), "Id max /A" ("VAR2 Name"), "Id min /A" ("VAR2 Name"), "Absolute plunger position" ("VAR2 Name")) -> (w93:string[])
    n385 = Array To Spreadsheet String(array=w64, 3:"" ("format string")) -> (spreadsheet string=w69:string)  [unwired: 1 in]
    n386 = Transpose 2D Array(2D array=w86) -> (transposed array=w85:dbl[][])
    n387 = String To Path(string=w63) -> (path=w60:path)
    n388 = Concatenate Strings(w59, "Prefix (time data)", "Suffix (time data)") -> (w101:string)
    n389 = Array To Spreadsheet String(array=w93, 3:"" ("format string")) -> (spreadsheet string=w92:string)  [unwired: 1 in]
    n390 = Array To Spreadsheet String(array=w85, 3:"%e" ("format string")) -> (spreadsheet string=w91:string)  [unwired: 1 in]
    n391 = String To Path(string=w101) -> (path=w100:path)
    n392 = local write "Serial port data"(w69) -> ()
    n393 = Write to Text File(file (use dialog)=w60, text=w64, error in=w58) -> (refnum out=w65:refnum<file>, error out=w66:errorcluster)  [unwired: 1 in, 1 out]
    n394 = Build Array(w92, w91) -> (w90:string[])
    n395 = Close File(refnum=w65, error in=w66) -> (error out=w57:errorcluster)  [unwired: 1 out]
    n396 = Write to Text File(file (use dialog)=w100, text=w90, error in=w57) -> (refnum out=w102:refnum<file>, error out=w89:errorcluster)  [unwired: 1 in, 1 out]
    n397 = Close File(refnum=w102, error in=w89) -> (error out=w83:errorcluster)  [unwired: 1 out]
  }
  "error out" <- w9
